vi "SCMP - Main Program v2.vi"() -> ()   [LabVIEW 2014]
doc: "Goodrich Exposure Range: .05microseconds to 798.9ms\n\nLow Gain (110e-/ADU)\nHigh Gain (6.5 e-/ADU)\n\nGA1280J Trigger Modes\n0 : Internally triggered; Internally timed\n1 : Externally triggered; Internally timed\n2 : Externally triggered; Externally timed\n3 : Externally gated; Internally timed\n\nFor list of camera commands\nsee Appendix A in the manual\n\n\nUse this template to build a standard state machine design pattern. Each state executes code and determines which state to transition to. Contrast this design pattern with the User Interface Event Handler pattern, in which code executes in response to user actions. Contrast this design pattern also with the Queued Message Handler pattern, in which each message handling code can queue zero or more new messages.\nNote: This template does not contain the most recent programming guidelines recommended by National Instruments. For a complete, project-based implementation of the Standard State Machine pattern, use the Create Project dialog box instead of this template."
uses:
  Controls/Main Program States.ctl
  <vilib>/Utility/error.llb/DialogType.ctl
  Controls/SCD - Calibration Optics Filter Wheel.ctl
  Controls/SCD - EDT - Emission Line Filter Wheel.ctl
  Controls/CoMP-S Controls/Emission Line Filter Wheel.ctl
  Controls/CoMP-S Controls/Polarization Optics Filter Wheel.ctl
  Controls/Global demo.vi
  Controls/SCD - FITS Cluster.ctl
  AISAS/Controls/focus.ctl
  AISAS/Controls/Diffuser.ctl
  Controls/Globals.vi
  AISAS/Mech/AISAS Mech.lvclass
  c:/mhutar/SCMP/Ancillary/Watlow EZ-ZONE/Public/Watbus.dll
  Ancillary/Watlow EZ-ZONE/Public/Watbus.dll
  Controls/peripherals.ctl
  AISAS/Controls/motor.ctl
  Controls/Cameras select.ctl
  Controls/FITS Data type.ctl
  Controls/Cbk Data type.ctl
  Controls/Cookbook.ctl
  Controls/beaning.ctl
  Camera/Andor Neo Info.ctl
  PI/PI Control.ctl
  AISAS/Controls/Rotation.ctl
panel:
  in  "Comment":string="Test"
  in  "Observer":string="Observer"
  out "Instrument":string
  out "Main Loop":bool=TRUE
  out "Log Loop":bool=TRUE
  out "Program":bool=TRUE
  out "Version":string
  in  "AOI Width 2":i64=2560
  in  "AOI Height 2":i64=2160
  out "Latest Actions":string="\r"
  out "cbk name":string="automated_find_focus_656.cbk"
  out "Main Loop Error":errorcluster={"status"=TRUE, "code"=0, "source"=""}
  in  "Tab Control":T1(tab)
  out "Camera T Image Zoom":u16[][](graph)
  out "Histogram Graph 2":T2(graph)
  out "Timestamp 2":timestamp=timestamp(3507746192.5616717 s since 1904-01-01)
  out "Mean ADU 2":u32=7788 format="%.1f"
  out "Sharpness 2":dbl format="%.2f"
  out "Camera FITS file path 2":path
  out "Camera R Image":u16[][](graph)
  in  "PI cam3 (mm)":T3 min=0.1 max=21.0 step=0.1 format="%.1f"
  in  "PI cam2 (mm)":T3 min=0.1 max=27.0 step=0.1 format="%.1f"
  in  "Calibration Optics":T4
  in  "Size":dbl format="%.2f"
  in  "Focus":T5 min=70.0 max=152.0 format="%.2f"
  in  "Andover Filter Wheel":T6
  in  "Calibration Wheel":T7
  in  "Binning":T8
  in  "Save Data to FITS?":bool
  out "Histogram Graph":T2(graph)
  in  "Snap Images":bool
  in  "Live Preview (Andor)":bool
  in  "Exposure (s)":dbl=0.02 min=1e-05 max=10.0 step=0.001 format="%_3p"
  out "Timestamp":timestamp=timestamp(3507746192.5616717 s since 1904-01-01)
  in  "PI cam1 (mm)":T3 min=0.1 max=27.0 step=0.1 format="%.1f"
  out "Camera FITS file path":path
  in  "Emission Line Filters":T9
  in  "Set Filter Wheels":bool
  out "Mean ADU":u32=7788 format="%.1f"
  out "Sharpness":dbl format="%.2f"
  in  "Diffuser":T10=enum."In Beam"
  in  "Rotation [deg]":T11 min=0.0 max=360.0 step=1.0 format="%.1f"
  in  "Move AISAS Mechanisms":bool
  in  "Motors":bool=TRUE
  out "Camera Image":u16[][](graph)
  out "Camera T Image":u16[][](graph)
  in  "Andor Adv Settings":bool
  in  "Diffuser 2":T10=enum."In Beam"
  in  "Focus 2":T5 min=70.0 max=152.0 format="%.2f"
  in  "Rotation [deg] 2":T11 min=0.0 max=360.0 step=1.0 format="%.1f"
  in  "Size 2":dbl format="%.2f"
  in  "Save Data to FITS?":bool=TRUE
  out "Cookbook":T12=[{"Data Type"=enum."ACQUIRE DATA", "Arg 1"=0.0, "Arg 2"=0.0, "Arg 3"=path "", "Comments"=""}, {"Data Type"=enum."ACQUIRE DATA", "Arg 1"=0.0, "Arg 2"=0.0, "Arg 3"=path "", "Comments"=""}]
  out "FITS Path from Last Recipe Acquiring Data":path
  in  "Load Cookbook":bool
  in  "Run Cookbook":bool
  out "# of Recipes":i16
  out "Selected Cookbook":path
  out "Recipe Files":string[](array[string])
  in  "limit max FPS to:":dbl=10.0 min=0.1 max=49.0 step=1.0 format="%.1g"
  out "Continually Read Log File":string="20160903-07:42:55 Live Preview Images\n20160903-07:44:38 Program Terminated\n20160903-07:45:16 Program Started\n20160903-07:45:18 Snap Single Image\n20160903-07:45:27 Live Preview Images\n20160903-07:46:17 Calibration & Filter wheel position:\t8\t5\n20160903-07:46:35 Live Preview Images\n20160903-07:50:39 Live Preview Images\n20160903-07:51:54 Camera Moved to Positon:-18.00\n20160903-07:51:55 Snap Single Image\n20160903-07:52:37 Loaded Cookbook\tfind_focus_656.cbk\n20160903-07:53:52 Run Cookbook\tfind_focus_656.cbk\n20160903-07:53:52 Recipe#0-exposure-20ms.rcp\n20160903-07:53:52 Recipe#1-fw-656.rcp\n20160903-07:53:54 Recipe#2-cal-open.rcp\n20160903-07:53:56 Recipe#3-move-absolute-neg19.rcp\n20160903-07:53:56 Recipe#4-take_656_focus_image.rcp\n20160903-07:54:02 Recipe#5-move-relative-neg0pt25.rcp\n20160903-07:55:56 Program Started\n20160903-07:56:02 Camera Moved to Positon:-18.00\n20160903-07:56:03 Snap Single Image\n20160903-07:56:35 Camera Moved to Positon:-19.00\n20160903-07:56:37 Snap Single Image\n20160903-07:56:58 Camera Moved to Positon:-20.00\n20160903-07:57:02 Snap Single Image\n20160903-07:57:20 Camera Moved to Positon:-21.00\n20160903-07:57:23 Snap Single Image\n20160903-07:57:36 Camera Moved to Positon:-22.00\n20160903-07:57:37 Snap Single Image\n20160903-07:57:53 Camera Moved to Positon:-25.00\n20160903-07:57:57 Snap Single Image\n20160903-07:58:13 Camera Moved to Positon:-30.00\n20160903-07:58:17 Snap Single Image\n20160903-07:58:43 Camera Moved to Positon:-18.00\n20160903-07:58:44 Snap Single Image\n20160903-07:58:58 Camera Moved to Positon:-17.00\n20160903-07:59:00 Snap Single Image\n20160903-08:00:39 Calibration & Filter wheel position:\t7\t6\n20160903-08:00:48 Snap Single Image\n20160903-08:01:42 Camera Moved to Positon:-65.00\n20160903-08:01:47 Snap Single Image\n20160903-08:02:07 Camera Moved to Positon:-70.00\n20160903-08:02:10 Snap Single Image\n20160903-08:02:51 Camera Moved to Positon:-75.00\n20160903-08:02:53 Snap Single Image\n20160903-08:03:25 Calibration & Filter wheel position:\t7\t7\n20160903-08:03:37 Snap Single Image\n20160903-08:03:55 Camera Moved to Positon:-76.00\n20160903-08:04:01 Snap Single Image\n20160903-08:04:13 Camera Moved to Positon:-77.00\n20160903-08:04:14 Snap Single Image\n20160903-08:04:24 Camera Moved to Positon:-78.00\n20160903-08:04:26 Snap Single Image\n20160903-08:04:38 Camera Moved to Positon:-79.00\n20160903-08:04:39 Snap Single Image\n20160903-08:04:50 Camera Moved to Positon:-83.00\n20160903-08:04:52 Snap Single Image\n20160903-08:05:10 Camera Moved to Positon:-73.00\n20160903-08:05:11 Snap Single Image\n20160903-08:05:22 Camera Moved to Positon:-71.00\n20160903-08:05:24 Snap Single Image\n20160903-08:05:34 Camera Moved to Positon:-69.00\n20160903-08:05:35 Snap Single Image\n20160903-08:05:47 Camera Moved to Positon:-67.00\n20160903-08:05:48 Snap Single Image\n20160903-08:06:13 Calibration & Filter wheel position:\t7\t8\n20160903-08:07:06 Snap Single Image\n20160903-08:07:17 Camera Moved to Positon:-69.00\n20160903-08:07:18 Snap Single Image\n20160903-08:07:28 Camera Moved to Positon:-71.00\n20160903-08:07:30 Snap Single Image\n20160903-08:07:40 Camera Moved to Positon:-73.00\n20160903-08:07:43 Snap Single Image\n20160903-08:07:53 Camera Moved to Positon:-75.00\n20160903-08:07:55 Snap Single Image\n20160903-08:08:04 Camera Moved to Positon:-77.00\n20160903-08:08:06 Snap Single Image\n20160903-08:08:17 Camera Moved to Positon:-79.00\n20160903-08:08:28 Snap Single Image\n20160903-08:08:43 Camera Moved to Positon:-81.00\n20160903-08:08:46 Snap Single Image\n20160903-08:09:05 Calibration & Filter wheel position:\t7\t9\n20160903-08:09:48 Camera Moved to Positon:-100.00\n20160903-08:09:50 Snap Single Image\n20160903-08:10:09 Snap Single Image\n20160903-08:10:26 Camera Moved to Positon:-100.00\n20160903-08:10:35 Camera Moved to Positon:-100.00\n20160903-08:10:37 Snap Single Image\n20160903-08:10:54 Camera Moved to Positon:-100.00\n20160903-08:10:59 Program Terminated\n20160903-08:12:25 Program Started\n20160903-08:12:33 Camera Moved to Positon:-100.00\n20160903-08:12:38 Program Terminated\n20160903-08:13:25 Program Started\n20160903-08:13:30 Camera Moved to Positon:-100.00\n20160903-08:13:37 Program Terminated\n20160903-08:14:12 Program Started\n20160903-08:14:19 Camera Moved to Positon:-100.00\n20160903-08:14:22 Snap Single Image\n20160903-08:14:37 Calibration & Filter wheel position:\t7\t9\n20160903-08:14:45 Snap Single Image\n20160903-08:14:56 Camera Moved to Positon:-105.00\n20160903-08:14:57 Snap Single Image\n20160903-08:15:10 Camera Moved to Positon:-110.00\n20160903-08:15:11 Snap Single Image\n20160903-08:15:23 Camera Moved to Positon:-115.00\n20160903-08:15:27 Snap Single Image\n20160903-08:15:39 Camera Moved to Positon:-120.00\n20160903-08:15:40 Snap Single Image\n20160903-08:15:59 Snap Single Image\n20160903-08:16:10 Camera Moved to Positon:-115.00\n20160903-08:16:11 Snap Single Image\n20160903-08:16:21 Camera Moved to Positon:-110.00\n20160903-08:16:22 Snap Single Image\n20160903-08:16:33 Camera Moved to Positon:-105.00\n20160903-08:16:36 Snap Single Image\n20160903-08:16:49 Camera Moved to Positon:-100.00\n20160903-08:16:51 Snap Single Image\n20160903-08:17:03 Camera Moved to Positon:-95.00\n20160903-08:17:05 Snap Single Image\n20160903-08:17:16 Camera Moved to Positon:-90.00\n20160903-08:17:18 Snap Single Image\n20160903-08:17:46 Camera Moved to Positon:-85.00\n20160903-08:17:49 Snap Single Image\n20160903-08:18:00 Camera Moved to Positon:-80.00\n20160903-08:18:02 Snap Single Image\n20160903-08:18:40 Calibration & Filter wheel position:\t7\t4\n20160903-08:18:59 Camera Moved to Positon:-20.00\n20160903-08:19:11 Snap Single Image\n20160903-08:19:23 Camera Moved to Positon:-18.00\n20160903-08:19:25 Snap Single Image\n20160903-08:19:38 Camera Moved to Positon:-22.00\n20160903-08:19:39 Snap Single Image\n20160903-08:19:51 Camera Moved to Positon:-24.00\n20160903-08:19:52 Snap Single Image\n20160903-08:20:04 Calibration & Filter wheel position:\t7\t3\n20160903-08:20:11 Snap Single Image\n20160903-08:20:22 Camera Moved to Positon:-18.00\n20160903-08:20:24 Snap Single Image\n20160903-08:20:39 Camera Moved to Positon:-16.00\n20160903-08:20:40 Snap Single Image\n20160903-08:20:53 Camera Moved to Positon:-14.00\n20160903-08:20:56 Snap Single Image\n20160903-08:21:06 Camera Moved to Positon:-12.00\n20160903-08:21:07 Snap Single Image\n20160903-08:21:16 Camera Moved to Positon:-10.00\n20160903-08:21:24 Snap Single Image\n20160903-08:21:34 Camera Moved to Positon: -8.00\n20160903-08:21:36 Snap Single Image\n20160903-08:22:12 Camera Moved to Positon: -6.00\n20160903-08:22:21 Snap Single Image\n20160903-08:23:09 Calibration & Filter wheel position:\t7\t1\n20160903-08:23:17 Snap Single Image\n20160903-08:23:27 Camera Moved to Positon: -4.00\n20160903-08:23:29 Snap Single Image\n20160903-08:23:37 Camera Moved to Positon: -2.00\n20160903-08:23:38 Snap Single Image\n20160903-08:23:47 Camera Moved to Positon:  0.00\n20160903-08:23:50 Snap Single Image\n20160903-08:26:00 Camera Moved to Positon:-18.00\n20160903-08:26:44 Program Started\n20160903-08:26:59 Camera Moved to Positon:-18.00\n20160903-08:27:05 Loaded Cookbook\tfind_focus_656.cbk\n20160903-08:27:12 Run Cookbook\tfind_focus_656.cbk\n20160903-08:27:12 Recipe#0-exposure-20ms.rcp\n20160903-08:27:12 Recipe#1-fw-656.rcp\n20160903-08:27:14 Recipe#2-cal-open.rcp\n20160903-08:27:16 Recipe#3-take_656_focus_image.rcp\n20160903-08:29:11 Camera Moved to Positon:-19.00\n20160903-08:29:17 Run Cookbook\tfind_focus_656.cbk\n20160903-08:29:17 Recipe#0-exposure-20ms.rcp\n20160903-08:29:17 Recipe#1-fw-656.rcp\n20160903-08:29:19 Recipe#2-cal-open.rcp\n20160903-08:29:21 Recipe#3-take_656_focus_image.rcp\n20160903-08:29:59 Camera Moved to Positon:-20.00\n20160903-08:30:03 Run Cookbook\tfind_focus_656.cbk\n20160903-08:30:03 Recipe#0-exposure-20ms.rcp\n20160903-08:30:03 Recipe#1-fw-656.rcp\n20160903-08:30:05 Recipe#2-cal-open.rcp\n20160903-08:30:07 Recipe#3-take_656_focus_image.rcp\n20160903-08:30:28 Camera Moved to Positon:-21.00\n20160903-08:30:32 Run Cookbook\tfind_focus_656.cbk\n20160903-08:30:32 Recipe#0-exposure-20ms.rcp\n20160903-08:30:32 Recipe#1-fw-656.rcp\n20160903-08:30:34 Recipe#2-cal-open.rcp\n20160903-08:30:36 Recipe#3-take_656_focus_image.rcp\n20160903-08:31:03 Camera Moved to Positon:-22.00\n20160903-08:31:06 Run Cookbook\tfind_focus_656.cbk\n20160903-08:31:06 Recipe#0-exposure-20ms.rcp\n20160903-08:31:06 Recipe#1-fw-656.rcp\n20160903-08:31:08 Recipe#2-cal-open.rcp\n20160903-08:31:10 Recipe#3-take_656_focus_image.rcp\n20160903-08:31:33 Camera Moved to Positon:-23.00\n20160903-08:31:38 Run Cookbook\tfind_focus_656.cbk\n20160903-08:31:38 Recipe#0-exposure-20ms.rcp\n20160903-08:31:38 Recipe#1-fw-656.rcp\n20160903-08:31:40 Recipe#2-cal-open.rcp\n20160903-08:31:42 Recipe#3-take_656_focus_image.rcp\n20160903-08:32:05 Camera Moved to Positon:-24.00\n20160903-08:32:08 Run Cookbook\tfind_focus_656.cbk\n20160903-08:32:08 Recipe#0-exposure-20ms.rcp\n20160903-08:32:08 Recipe#1-fw-656.rcp\n20160903-08:32:10 Recipe#2-cal-open.rcp\n20160903-08:32:12 Recipe#3-take_656_focus_image.rcp\n20160903-08:32:35 Camera Moved to Positon:-25.00\n20160903-08:32:40 Run Cookbook\tfind_focus_656.cbk\n20160903-08:32:40 Recipe#0-exposure-20ms.rcp\n20160903-08:32:40 Recipe#1-fw-656.rcp\n20160903-08:32:42 Recipe#2-cal-open.rcp\n20160903-08:32:44 Recipe#3-take_656_focus_image.rcp\n20160903-08:33:03 Camera Moved to Positon:-26.00\n20160903-08:33:07 Run Cookbook\tfind_focus_656.cbk\n20160903-08:33:07 Recipe#0-exposure-20ms.rcp\n20160903-08:33:07 Recipe#1-fw-656.rcp\n20160903-08:33:09 Recipe#2-cal-open.rcp\n20160903-08:33:11 Recipe#3-take_656_focus_image.rcp\n20160903-08:33:32 Camera Moved to Positon:-27.00\n20160903-08:33:34 Run Cookbook\tfind_focus_656.cbk\n20160903-08:33:34 Recipe#0-exposure-20ms.rcp\n20160903-08:33:34 Recipe#1-fw-656.rcp\n20160903-08:33:36 Recipe#2-cal-open.rcp\n20160903-08:33:38 Recipe#3-take_656_focus_image.rcp\n20160903-08:34:01 Camera Moved to Positon:-28.00\n20160903-08:34:05 Run Cookbook\tfind_focus_656.cbk\n20160903-08:34:05 Recipe#0-exposure-20ms.rcp\n20160903-08:34:05 Recipe#1-fw-656.rcp\n20160903-08:34:07 Recipe#2-cal-open.rcp\n20160903-08:34:09 Recipe#3-take_656_focus_image.rcp\n20160903-08:36:44 Camera Moved to Positon:-85.00\n20160903-08:36:51 Loaded Cookbook\tfind_focus_1083.cbk\n20160903-08:37:11 Loaded Cookbook\tfind_focus_1083.cbk\n20160903-08:37:20 Run Cookbook\tfind_focus_1083.cbk\n20160903-08:37:20 Recipe#0-exposure-120ms.rcp\n20160903-08:37:20 Recipe#1-fw-1083.rcp\n20160903-08:37:22 Recipe#2-cal-open.rcp\n20160903-08:37:23 Recipe#3-take_1083_focus_image.rcp\n20160903-08:38:05 Camera Moved to Positon:-86.00\n20160903-08:38:11 Run Cookbook\tfind_focus_1083.cbk\n20160903-08:38:11 Recipe#0-exposure-120ms.rcp\n20160903-08:38:11 Recipe#1-fw-1083.rcp\n20160903-08:38:13 Recipe#2-cal-open.rcp\n20160903-08:38:15 Recipe#3-take_1083_focus_image.rcp\n20160903-08:38:39 Camera Moved to Positon:-87.00\n20160903-08:38:43 Run Cookbook\tfind_focus_1083.cbk\n20160903-08:38:43 Recipe#0-exposure-120ms.rcp\n20160903-08:38:43 Recipe#1-fw-1083.rcp\n20160903-08:38:45 Recipe#2-cal-open.rcp\n20160903-08:38:47 Recipe#3-take_1083_focus_image.rcp\n20160903-08:39:05 Camera Moved to Positon:-88.00\n20160903-08:39:09 Run Cookbook\tfind_focus_1083.cbk\n20160903-08:39:10 Recipe#0-exposure-120ms.rcp\n20160903-08:39:10 Recipe#1-fw-1083.rcp\n20160903-08:39:12 Recipe#2-cal-open.rcp\n20160903-08:39:13 Recipe#3-take_1083_focus_image.rcp\n20160903-08:43:45 Snap Single Image\n20160903-08:43:56 Run Cookbook\tfind_focus_1083.cbk\n20160903-08:43:56 Recipe#0-exposure-120ms.rcp\n20160903-08:43:56 Recipe#1-fw-1083.rcp\n20160903-08:43:58 Recipe#2-cal-open.rcp\n20160903-08:44:00 Recipe#3-take_1083_focus_image.rcp\n20160903-08:44:24 Camera Moved to Positon:-90.00\n20160903-08:44:32 Camera Moved to Positon:-89.00\n20160903-08:44:36 Run Cookbook\tfind_focus_1083.cbk\n20160903-08:44:36 Recipe#0-exposure-120ms.rcp\n20160903-08:44:36 Recipe#1-fw-1083.rcp\n20160903-08:44:38 Recipe#2-cal-open.rcp\n20160903-08:44:40 Recipe#3-take_1083_focus_image.rcp\n20160903-08:45:03 Camera Moved to Positon:-90.00\n20160903-08:45:11 Run Cookbook\tfind_focus_1083.cbk\n20160903-08:45:12 Recipe#0-exposure-120ms.rcp\n20160903-08:45:12 Recipe#1-fw-1083.rcp\n20160903-08:45:14 Recipe#2-cal-open.rcp\n20160903-08:45:15 Recipe#3-take_1083_focus_image.rcp\n20160903-08:45:38 Camera Moved to Positon:-91.00\n20160903-08:45:41 Run Cookbook\tfind_focus_1083.cbk\n20160903-08:45:41 Recipe#0-exposure-120ms.rcp\n20160903-08:45:42 Recipe#1-fw-1083.rcp\n20160903-08:45:43 Recipe#2-cal-open.rcp\n20160903-08:45:45 Recipe#3-take_1083_focus_image.rcp\n20160903-08:46:07 Camera Moved to Positon:-92.00\n20160903-08:46:12 Run Cookbook\tfind_focus_1083.cbk\n20160903-08:46:12 Recipe#0-exposure-120ms.rcp\n20160903-08:46:12 Recipe#1-fw-1083.rcp\n20160903-08:46:14 Recipe#2-cal-open.rcp\n20160903-08:46:16 Recipe#3-take_1083_focus_image.rcp\n20160903-08:46:53 Camera Moved to Positon:-93.00\n20160903-08:46:56 Run Cookbook\tfind_focus_1083.cbk\n20160903-08:46:56 Recipe#0-exposure-120ms.rcp\n20160903-08:46:56 Recipe#1-fw-1083.rcp\n20160903-08:46:58 Recipe#2-cal-open.rcp\n20160903-08:47:00 Recipe#3-take_1083_focus_image.rcp\n20160903-08:48:13 Calibration & Filter wheel position:\t7\t3\n20160903-08:51:11 Camera Moved to Positon:-10.00\n20160903-08:51:19 Camera Moved to Positon: -5.00\n20160903-08:51:20 Live Preview Images\n20160903-08:51:43 Loaded Cookbook\tfind_focus_589.cbk\n20160903-08:52:08 Loaded Cookbook\tfocus-656.cbk\n20160903-08:52:09 Run Cookbook\tfocus-656.cbk\n20160903-08:52:09 Recipe#0-fw-656.rcp\n20160903-08:52:11 Recipe#1-cal-clear.rcp\n20160903-08:52:13 Recipe#2-exposure-200ms.rcp\n20160903-08:52:13 Recipe#3-focus-656.rcp\n20160903-08:52:24 Program Started\n20160903-08:52:33 Loaded Cookbook\tfocus-656.cbk\n20160903-08:52:40 Camera Moved to Positon: -5.00\n20160903-08:52:46 Loaded Cookbook\tfind_focus_589.cbk\n20160903-08:52:48 Run Cookbook\tfind_focus_589.cbk\n20160903-08:52:48 Recipe#0-exposure-20ms.rcp\n20160903-08:52:48 Recipe#1-fw-589.rcp\n20160903-08:52:50 Recipe#2-cal-open.rcp\n20160903-08:52:52 Recipe#3-take_589_focus_image.rcp\n20160903-08:54:55 Run Cookbook\tfind_focus_589.cbk\n20160903-08:54:55 Recipe#0-exposure-20ms.rcp\n20160903-08:54:56 Recipe#1-fw-589.rcp\n20160903-08:54:57 Recipe#2-cal-open.rcp\n20160903-08:54:59 Recipe#3-take_589_focus_image.rcp\n20160903-08:55:19 Live Preview Images\n20160903-08:56:01 Camera Moved to Positon: -6.00\n20160903-08:56:04 Run Cookbook\tfind_focus_589.cbk\n20160903-08:56:04 Recipe#0-exposure-20ms.rcp\n20160903-08:56:04 Recipe#1-fw-589.rcp\n20160903-08:56:06 Recipe#2-cal-open.rcp\n20160903-08:56:08 Recipe#3-take_589_focus_image.rcp\n20160903-08:56:40 Camera Moved to Positon: -7.00\n20160903-08:58:30 Run Cookbook\tfind_focus_589.cbk\n20160903-08:58:30 Recipe#0-exposure-20ms.rcp\n20160903-08:58:30 Recipe#1-fw-589.rcp\n20160903-08:58:32 Recipe#2-cal-open.rcp\n20160903-08:58:34 Recipe#3-take_589_focus_image.rcp\n20160903-08:59:22 Camera Moved to Positon: -8.00\n20160903-09:14:18 Program Terminated\n20160903-09:40:55 Program Started\n20160903-09:44:03 Loaded Cookbook\tautomated_find_focus_656.cbk\n20160903-09:44:43 Loaded Cookbook\tautomated_find_focus_656.cbk\n20160903-09:44:57 Run Cookbook\tautomated_find_focus_656.cbk\n20160903-09:44:57 Recipe#0-exposure-20ms.rcp\n20160903-09:44:57 Recipe#1-fw-656.rcp\n20160903-09:44:59 Recipe#2-cal-open.rcp\n20160903-09:45:01 Recipe#3-move-absolute-neg15.rcp\n20160903-09:45:02 Recipe#4-take_656_focus_image.rcp\n20160903-09:45:16 Recipe#5-move-relative-neg0pt25.rcp\n20160903-09:45:17 Recipe#6-take_656_focus_image.rcp\n20160903-09:45:31 Recipe#7-move-relative-neg0pt25.rcp\n20160903-09:45:32 Recipe#8-take_656_focus_image.rcp\n20160903-09:45:46 Recipe#9-move-relative-neg0pt25.rcp\n20160903-09:45:47 Recipe#10-take_656_focus_image.rcp\n20160903-09:46:01 Recipe#11-move-relative-neg0pt25.rcp\n20160903-09:46:02 Recipe#12-take_656_focus_image.rcp\n20160903-09:46:17 Recipe#13-move-relative-neg0pt25.rcp\n20160903-09:46:18 Recipe#14-take_656_focus_image.rcp\n20160903-09:46:32 Recipe#15-move-relative-neg0pt25.rcp\n20160903-09:46:33 Recipe#16-take_656_focus_image.rcp\n20160903-09:46:47 Recipe#17-move-relative-neg0pt25.rcp\n20160903-09:46:48 Recipe#18-take_656_focus_image.rcp\n20160903-09:47:02 Recipe#19-move-relative-neg0pt25.rcp\n20160903-09:47:03 Recipe#20-take_656_focus_image.rcp\n20160903-09:47:17 Recipe#21-move-relative-neg0pt25.rcp\n20160903-09:47:17 Recipe#22-take_656_focus_image.rcp\n20160903-09:47:32 Recipe#23-move-relative-neg0pt25.rcp\n20160903-09:47:32 Recipe#24-take_656_focus_image.rcp\n20160903-09:47:46 Recipe#25-move-relative-neg0pt25.rcp\n20160903-09:47:47 Recipe#26-take_656_focus_image.rcp\n20160903-09:48:02 Recipe#27-move-relative-neg0pt25.rcp\n20160903-09:48:03 Recipe#28-take_656_focus_image.rcp\n20160903-09:48:17 Recipe#29-move-relative-neg0pt25.rcp\n20160903-09:48:17 Recipe#30-take_656_focus_image.rcp\n20160903-09:48:32 Recipe#31-move-relative-neg0pt25.rcp\n20160903-09:48:33 Recipe#32-take_656_focus_image.rcp\n20160903-09:48:49 Recipe#33-move-relative-neg0pt25.rcp\n20160903-09:48:49 Recipe#34-take_656_focus_image.rcp\n20160903-09:49:05 Recipe#35-move-relative-neg0pt25.rcp\n20160903-09:49:06 Recipe#36-take_656_focus_image.rcp\n20160903-09:49:23 Recipe#37-move-relative-neg0pt25.rcp\n20160903-09:49:24 Recipe#38-take_656_focus_image.rcp\n20160903-09:49:41 Recipe#39-move-relative-neg0pt25.rcp\n20160903-09:49:42 Recipe#40-take_656_focus_image.rcp\n20160903-09:50:01 Recipe#41-move-relative-neg0pt25.rcp\n20160903-09:50:01 Recipe#42-take_656_focus_image.rcp\n20160903-09:50:20 Recipe#43-move-relative-neg0pt25.rcp\n20160903-09:50:21 Recipe#44-take_656_focus_image.rcp\n20160903-09:54:36 Loaded Cookbook\tautomated_find_focus_656.cbk\n20160903-09:54:47 Loaded Cookbook\tautomated_find_focus_656.cbk\n20160903-09:55:40 Loaded Cookbook\tautomated_find_focus_656.cbk\n20160903-09:55:54 Run Cookbook\tautomated_find_focus_656.cbk\n20160903-09:55:54 Recipe#0-exposure-40ms.rcp\n20160903-09:55:54 Recipe#1-fw-656.rcp\n20160903-09:55:56 Recipe#2-cal-open.rcp\n20160903-09:55:58 Recipe#3-move-absolute-neg15.rcp\n20160903-09:55:59 Recipe#4-take_656_focus_image.rcp\n20160903-09:56:06 Recipe#5-move-relative-neg0pt5.rcp\n20160903-09:56:07 Recipe#6-take_656_focus_image.rcp\n20160903-09:56:14 Recipe#7-move-relative-neg0pt5.rcp\n20160903-09:56:15 Recipe#8-take_656_focus_image.rcp\n20160903-09:56:22 Recipe#9-move-relative-neg0pt5.rcp\n20160903-09:56:22 Recipe#10-take_656_focus_image.rcp\n20160903-09:56:29 Recipe#11-move-relative-neg0pt5.rcp\n20160903-09:56:30 Recipe#12-take_656_focus_image.rcp\n20160903-09:56:37 Recipe#13-move-relative-neg0pt5.rcp\n20160903-09:56:38 Recipe#14-take_656_focus_image.rcp\n20160903-09:56:45 Recipe#15-move-relative-neg0pt5.rcp\n20160903-09:56:45 Recipe#16-take_656_focus_image.rcp\n20160903-09:56:52 Recipe#17-move-relative-neg0pt5.rcp\n20160903-09:56:53 Recipe#18-take_656_focus_image.rcp\n20160903-09:57:00 Recipe#19-move-relative-neg0pt5.rcp\n20160903-09:57:01 Recipe#20-take_656_focus_image.rcp\n20160903-09:57:08 Recipe#21-move-relative-neg0pt5.rcp\n20160903-09:57:09 Recipe#22-take_656_focus_image.rcp\n20160903-09:57:16 Recipe#23-move-relative-neg0pt5.rcp\n20160903-09:57:16 Recipe#24-take_656_focus_image.rcp\n20160903-09:57:23 Recipe#25-move-relative-neg0pt5.rcp\n20160903-09:57:24 Recipe#26-take_656_focus_image.rcp\n20160903-09:57:31 Recipe#27-move-relative-neg0pt5.rcp\n20160903-09:57:32 Recipe#28-take_656_focus_image.rcp\n20160903-09:57:39 Recipe#29-move-relative-neg0pt5.rcp\n20160903-09:57:40 Recipe#30-take_656_focus_image.rcp\n20160903-09:57:47 Recipe#31-move-relative-neg0pt5.rcp\n20160903-09:57:48 Recipe#32-take_656_focus_image.rcp\n20160903-09:57:55 Recipe#33-move-relative-neg0pt5.rcp\n20160903-09:57:56 Recipe#34-take_656_focus_image.rcp\n20160903-09:58:03 Recipe#35-move-relative-neg0pt5.rcp\n20160903-09:58:03 Recipe#36-take_656_focus_image.rcp\n20160903-09:58:10 Recipe#37-move-relative-neg0pt5.rcp\n20160903-09:58:11 Recipe#38-take_656_focus_image.rcp\n20160903-09:58:18 Recipe#39-move-relative-neg0pt5.rcp\n20160903-09:58:19 Recipe#40-take_656_focus_image.rcp\n20160903-09:58:26 Recipe#41-move-relative-neg0pt5.rcp\n20160903-09:58:27 Recipe#42-take_656_focus_image.rcp\n20160903-09:58:34 Recipe#43-move-relative-neg0pt5.rcp\n20160903-09:58:35 Recipe#44-take_656_focus_image.rcp\n20160903-10:46:33 Program Terminated\n20160903-12:25:32 Program Started\n20160903-12:26:22 Program Terminated\n20160903-12:45:45 Program Started\n20160903-12:45:56 Program Terminated\n20160903-12:49:12 Program Started\n20160903-12:49:15 Loaded Cookbook\tautomated_find_focus_656.cbk\n20160903-12:49:24 Run Cookbook\tautomated_find_focus_656.cbk\n20160903-12:49:25 Recipe#0-exposure-40ms.rcp\n20160903-12:49:25 Recipe#1-fw-656.rcp\n20160903-12:49:26 Recipe#2-cal-open.rcp\n20160903-12:49:28 Recipe#3-move-absolute-neg15.rcp\n20160903-12:49:29 Recipe#4-take_656_focus_image.rcp\n20160903-12:49:32 Recipe#5-move-relative-neg0pt5.rcp\n20160903-12:49:33 Recipe#6-take_656_focus_image.rcp\n20160903-12:49:36 Recipe#7-move-relative-neg0pt5.rcp\n20160903-12:49:36 Recipe#8-take_656_focus_image.rcp\n20160903-12:49:39 Recipe#9-move-relative-neg0pt5.rcp\n20160903-12:49:40 Recipe#10-take_656_focus_image.rcp\n20160903-12:49:43 Recipe#11-move-relative-neg0pt5.rcp\n20160903-12:49:43 Recipe#12-take_656_focus_image.rcp\n20160903-12:49:46 Recipe#13-move-relative-neg0pt5.rcp\n20160903-12:49:47 Recipe#14-take_656_focus_image.rcp\n20160903-12:49:49 Recipe#15-move-relative-neg0pt5.rcp\n20160903-12:49:50 Recipe#16-take_656_focus_image.rcp\n20160903-12:49:53 Recipe#17-move-relative-neg0pt5.rcp\n20160903-12:49:53 Recipe#18-take_656_focus_image.rcp\n20160903-12:49:56 Recipe#19-move-relative-neg0pt5.rcp\n20160903-12:49:57 Recipe#20-take_656_focus_image.rcp\n20160903-12:49:59 Recipe#21-move-relative-neg0pt5.rcp\n20160903-12:50:00 Recipe#22-take_656_focus_image.rcp\n20160903-12:50:03 Recipe#23-move-relative-neg0pt5.rcp\n20160903-12:50:04 Recipe#24-take_656_focus_image.rcp\n20160903-12:50:06 Recipe#25-move-relative-neg0pt5.rcp\n20160903-12:50:07 Recipe#26-take_656_focus_image.rcp\n20160903-12:50:10 Recipe#27-move-relative-neg0pt5.rcp\n20160903-12:50:10 Recipe#28-take_656_focus_image.rcp\n20160903-12:50:13 Recipe#29-move-relative-neg0pt5.rcp\n20160903-12:50:14 Recipe#30-take_656_focus_image.rcp\n20160903-12:50:16 Recipe#31-move-relative-neg0pt5.rcp\n20160903-12:50:17 Recipe#32-take_656_focus_image.rcp\n20160903-12:50:20 Recipe#33-move-relative-neg0pt5.rcp\n20160903-12:50:20 Recipe#34-take_656_focus_image.rcp\n20160903-12:50:23 Recipe#35-move-relative-neg0pt5.rcp\n20160903-12:50:24 Recipe#36-take_656_focus_image.rcp\n20160903-12:50:26 Recipe#37-move-relative-neg0pt5.rcp\n20160903-12:50:27 Recipe#38-take_656_focus_image.rcp\n20160903-12:50:30 Recipe#39-move-relative-neg0pt5.rcp\n20160903-12:50:31 Recipe#40-take_656_focus_image.rcp\n20160903-12:50:33 Recipe#41-move-relative-neg0pt5.rcp\n20160903-12:50:34 Recipe#42-take_656_focus_image.rcp\n20160903-12:50:37 Recipe#43-move-relative-neg0pt5.rcp\n20160903-12:50:37 Recipe#44-take_656_focus_image.rcp\n20160903-13:54:17 Program Terminated\n20160903-14:07:18 Program Started\n20160903-14:08:12 Program Terminated\n20160903-14:20:46 Program Started\n20160903-14:22:56 Program Terminated\n20160903-14:23:20 Program Started\n20160903-14:25:03 Program Terminated\n20160903-14:31:16 Program Started\n20160903-14:32:59 Program Terminated\n20160903-14:33:26 Program Started\n20160903-14:35:01 Program Terminated\n20160903-14:36:43 Program Started\n20160903-14:38:01 Program Terminated\n20160903-14:39:22 Program Started\n20160903-14:39:47 Program Terminated\n20160903-14:40:22 Program Started\n20160903-14:41:59 Program Terminated\n20160903-15:07:40 Program Started\n20160903-15:10:18 Program Terminated\n20160903-15:19:59 Program Started\n20160903-15:20:17 Program Terminated\n20160903-15:20:43 Program Started\n20160903-15:20:43 Program Terminated\n20160903-15:21:33 Program Started\n20160903-15:22:45 Program Terminated\n20160903-15:24:43 Program Started\n20160903-15:26:40 Program Terminated\n20160903-15:29:07 Program Started\n20160903-15:29:52 Loaded Cookbook\tautomated_find_focus_656.cbk\n20160903-15:30:08 Loaded Cookbook\tautomated_find_focus_656.cbk\n"
  out "min Cookbook Exposure [s]":dbl=200.0 format="%#_3p"
  out "Today's SCMP Log File":path
  out "Cookbook Comments":string
  in  "Mod/Seq":bool
  in  "Enable Data Logging":bool=TRUE
  out "Today's SCMP Eng  File":path
  out "Air around \nprefilter wheel [C]":sgl(graph)
  out "Lyot Filter Temp [C]":dbl(graph)
  out "Air around Camera [C]":sgl(graph)
  out "Air around Lyot Filter [C]":dbl(graph)
  out "Eng Data Error":errorcluster={"status"=TRUE, "code"=0, "source"=""}
  out "Camera 1 Temp [C}":dbl(graph)=-21.03
  out "Camera 2 Temp [C}":dbl(graph)=-21.03
  out "FITS Header":T14={"Wavelength (nm)"=530.15, "Exposure (s)"=0.05, "Tuning Delay (ms)"=1000.0, "Beam Type (-1/1)"=1.0, "Tuning Voltages"=[1.111, 2.222, 3.333, 4.444], "Observer"="observer", "Light Shapping Diffuser"=enum."In Beam", "Comment"="", "Data Type"=9, "Mod Cycles"=0, "SCD Calibration Optics"=enum."1 - Polarizer @0, I+Q", "SCD Emission Line Filter"=enum."1-557.6nm", "Cookbook"="", "COMP-S Calibration Wheel"=enum."Dark", "COMP-S Andover Filter Wheel"=enum."530.3nm/HWB 0.34nm (Fe XIV)", "FOV Rotation (deg)"=66.0, "Objective Lens Position (mm)"=0.0, "Occulter size"=0.0, "Time End"=timestamp(3382374145.421875 s since 1904-01-01), "Acc Exposure (s)"=0.0, "Time Stamp Array"=[], "Camera Serial Number"=[], "Camera Temp"=[], "Camera PI (mm)"=[], "Time Start"=timestamp(3382374145.421875 s since 1904-01-01), "Peripherals"={"ILX controler"=FALSE, "Zone temperatures"=FALSE, "Andor"=FALSE, "Andor 2"=FALSE, "PI Stages"=FALSE, "AISAS mechanisms"=FALSE, "AISAS Mech.lvclass"=refnum, "Zone temp ref"=variant, "FWs"=FALSE}, "FITS paths"=[], "Cameras"=enum."Andor", "load preset cbk"=FALSE, "periodic check count"=0, "COMP-S Calibration Wheel 2"=enum."Dark", "Calib"=enum."Dark", "Abso Aperture"=40.0, "Nominal Aperture"=196.0} {"Nominal Aperture" format="%.1f"; "Abso Aperture" format="%.1f"; "Camera PI (mm)" format="%_3g"; "Acc Exposure (s)" format="%^.3g"; "Occulter size" format="%.2f"; "Objective Lens Position (mm)" min=70.0 max=152.0 format="%.2f"; "FOV Rotation (deg)" format="%.1f"; "Data Type" items=["LIVE", "DARK", "FLAT", "CALI", "OBSE", "ABSO", "AURE", "TARG", "OBJE", "HOLE", "OREX", "THRO", "CHIP"]; "Exposure (s)" format="%^.3g"; "Wavelength (nm)" format="%_6g"}
  out "Andor Neo":T17[](array[typedef]) {"Exposure (s)" format="%^.3g"; "Time at Synch" format="%<%H:%M:%S>T"; "Interframe Time" format="%#_3g"; "Frame Readout Time" format="%_3g"; "Row Readout Time" format="%_3g"}
  in  "Stop":bool=TRUE
  # "Filter Wheels"
  # "Camera Settings"
  # "AISAS mechanisms"
  # "Occulter"
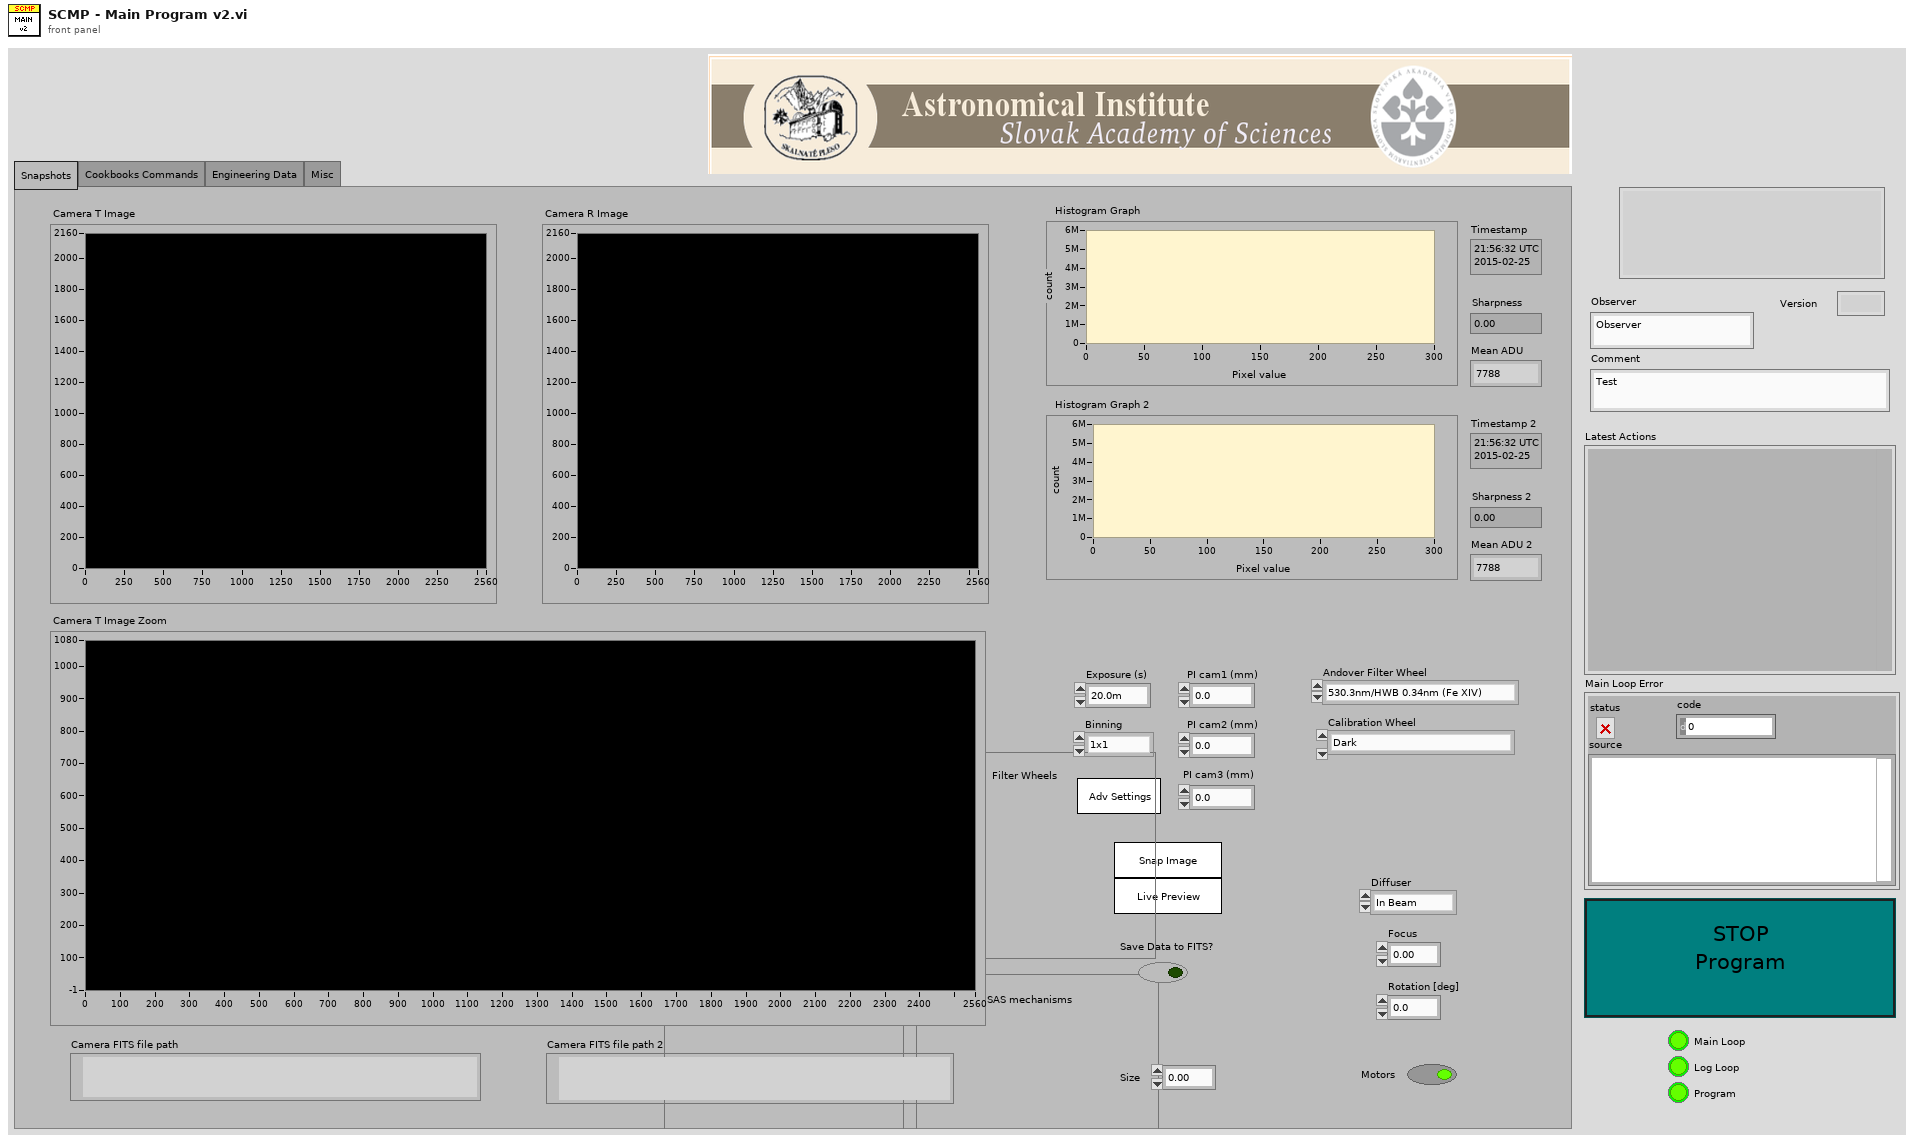
[diagram p1: front panel]
types:
  T1 = enum32{"Snapshots", "Cookbooks Commands", "Engineering Data", "Misc"}
  T2 = cluster{"X Values":dbl[], "Histogram: h(x)":i32[]}
  T3 = typedef "PI Control.ctl" = dbl
  T4 = typedef "SCD - Calibration Optics Filter Wheel.ctl" = enum16{"1 - Polarizer @0, I+Q", "2 - Polarizer @90, I-Q", "3 - Polarizer @45, I+U", "4 - Polarizer @135, I-U", "5 - Polarizer @0, Retarder @45, I+V", "6 - Polarizer @0, Retarder @135, I-V", "7 - Dark", "8 - Clear", "9 - N/A"}
  T5 = typedef "focus.ctl" = dbl
  T6 = typedef "Emission Line Filter Wheel.ctl" = enum16{"530.3nm/HWB 0.34nm (Fe XIV)", "587.6nm/HBW 0.44nm (He I D3)", "637.5nm/HBW 0.53nm (Fe X)", "656.3nm/HBW 0.57nm (H-Alpha)", "789.2nm/HBW 0.85nm (Fe XI)", "854.2nm/HBW 1.01nm (Ca I)", "1074.7nm/HBW 2.34nm (Fe XIII)", "1079.8nm/HBW 1.64nm (Fe XIII)", "1083.0nm/HBW 1.66nm (He I)"}
  T7 = typedef "Polarization Optics Filter Wheel.ctl" = enum16{"Dark", "Clear", "Exchange Lens", "Polarizer @0, I+Q", "Polarizer @90, I-Q", "Polarizer @45, I+U", "Polarizer @135, I-U", "Polarizer @0, Retarder @45, I+V", "Polarizer @0, Retarder @135, I-V"}
  T8 = typedef "beaning.ctl" = enum16{"1x1", "2x2", "3x3", "4x4", "8x8"}
  T9 = typedef "SCD - EDT - Emission Line Filter Wheel.ctl" = enum16{"1-557.6nm", "2-587.6nm", "3-589.6nm", "4-630.2nm", "5-656.4nm", "6-849.8nm", "7-854.2nm", "8-866.2nm", "9-1083.0nm"}
  T10 = typedef "Diffuser.ctl" = enum16{"Out of Beam", "In Beam"}
  T11 = typedef "Rotation.ctl" = dbl
  T12 = typedef "Cookbook.ctl" = cluster{"Data Type":T13, "Arg 1":sgl, "Arg 2":sgl, "Arg 3":path, "Comments":string}[]
  T13 = typedef "Cbk Data type.ctl" = enum32{"ACQUIRE DATA", "SET DIFFUSER", "CAL-FW", "WAVELENGTH-FW", "INSTR. ROTATION", "SET FOCUS", "DATATYPE", "SET EXPOSURE", "CBK COMMENTS", "MOVE-PI", "MOVE-PI2", "MOVE-PI3", "DWELL TIME", "BINNING"}
  T14 = typedef "SCD - FITS Cluster.ctl" = cluster{"Wavelength (nm)":dbl, "Exposure (s)":dbl, "Tuning Delay (ms)":dbl, "Beam Type (-1/1)":dbl, "Tuning Voltages":dbl[], "Observer":string, "Light Shapping Diffuser":T10, "Comment":string, "Data Type":u16, "Mod Cycles":u16, "SCD Calibration Optics":T4, "SCD Emission Line Filter":T9, "Cookbook":string, "COMP-S Calibration Wheel":T7, "COMP-S Andover Filter Wheel":T6, "FOV Rotation (deg)":dbl, "Objective Lens Position (mm)":T5, "Occulter size":dbl, "Time End":timestamp, "Acc Exposure (s)":dbl, "Time Stamp Array":timestamp[], "Camera Serial Number":string[], "Camera Temp":dbl[], "Camera PI (mm)":dbl[], "Time Start":timestamp, "Peripherals":T15, "FITS paths":path[], "Cameras":T16, "load preset cbk":bool, "periodic check count":i32, "COMP-S Calibration Wheel 2":T7, "Calib":enum16{"Dark", "Flat"}, "Abso Aperture":dbl, "Nominal Aperture":dbl}
  T15 = typedef "peripherals.ctl" = cluster{"ILX controler":bool, "Zone temperatures":bool, "Andor":bool, "Andor 2":bool, "PI Stages":bool, "AISAS mechanisms":bool, "AISAS Mech.lvclass":refnum<class "AISAS Mech.lvclass">, "Zone temp ref":variant, "FWs":bool}
  T16 = typedef "Cameras select.ctl" = enum16{"Andor", "GDR"}
  T17 = typedef "Andor Neo Info.ctl" = cluster{"Handle":i32, "Pixel Encoding":string, "AOI Width":i32, "AOI Height":i32, "AOI Stride":i32, "Row Readout Time":dbl, "Frame Readout Time":dbl, "Interframe Time":dbl, "Semaphore":T18, "SerialNumber":string, "Camera Model":string, "Controller ID":string, "Firmware Version":string, "Shutter":string, "BDiv":u8, "Time at Synch":timestamp, "Idx":i32, "PreAmp":string, "Binning":T8, "PixelReadoutRate":string, "Exposure (s)":dbl, "Image Bytes":i64, "Image Pixels":i64, "SpuriousNoiseFilter":bool, "Overlap":bool, "CycleMode":string}
  T18 = typedef "Semaphore RefNum" = refnum<k1>
  T19 = typedef "Main Program States.ctl" = enum16{"Initialize", "Wait for Event", "Periodic Check", "Update UI", "Update Camera UI", "Load Cookbook", "Run Cookbook", "Snap Images", "Live Preview", "Set Filter Wheel", "Set Calibration Wheel", "AISAS Motors on/off", "AISAS Move", "Move AISAS Mechanisms", "Stop", "Change Camera Exposure", "Change Camera Stage Position", "Set Camera AOI", "Andor Adv Settings", "Update Image", "Run Dark", "Calib acq", "Process Calib"}
  T20 = typedef "SCD - FITS Cluster.ctl" = cluster{"Wavelength (nm)":dbl, "Exposure (s)":dbl, "Tuning Delay (ms)":dbl, "Beam Type (-1/1)":dbl, "Tuning Voltages":dbl[], "Observer":string, "Light Shapping Diffuser":T10, "Comment":string, "Data Type":T21, "Mod Cycles":u16, "SCD Calibration Optics":T4, "SCD Emission Line Filter":T9, "Cookbook":string, "COMP-S Calibration Wheel":T7, "COMP-S Andover Filter Wheel":T6, "FOV Rotation (deg)":dbl, "Objective Lens Position (mm)":T5, "Occulter size":dbl, "Time End":timestamp, "Acc Exposure (s)":dbl, "Time Stamp Array":timestamp[], "Camera Serial Number":string[], "Camera Temp":dbl[], "Camera PI (mm)":dbl[], "Time Start":timestamp, "Peripherals":T15, "FITS paths":path[], "Cameras":T16, "load preset cbk":bool, "periodic check count":i32, "COMP-S Calibration Wheel 2":T7, "Calib":enum16{"Dark", "Flat"}, "Abso Aperture":dbl, "Nominal Aperture":dbl, "Pointer IP":string}
  T21 = typedef "FITS Data type.ctl" = enum16{"LIVE", "DARK", "FLAT", "CALI", "OBSE", "ABSO", "AURE", "TARG", "OBJE", "HOLE", "OREX", "THRO", "CHIP"}
  T22 = enum8{"Enabled", "Disabled", "Disabled and Grayed Out"}
  T23 = typedef "motor.ctl" = enum32{"Rotation", "Diffuser ", "Focus"}
  T24 = enum16{"Emission Line Filters", "Calibration Polarizers"}
  T25 = typedef "DialogType.ctl" = u16
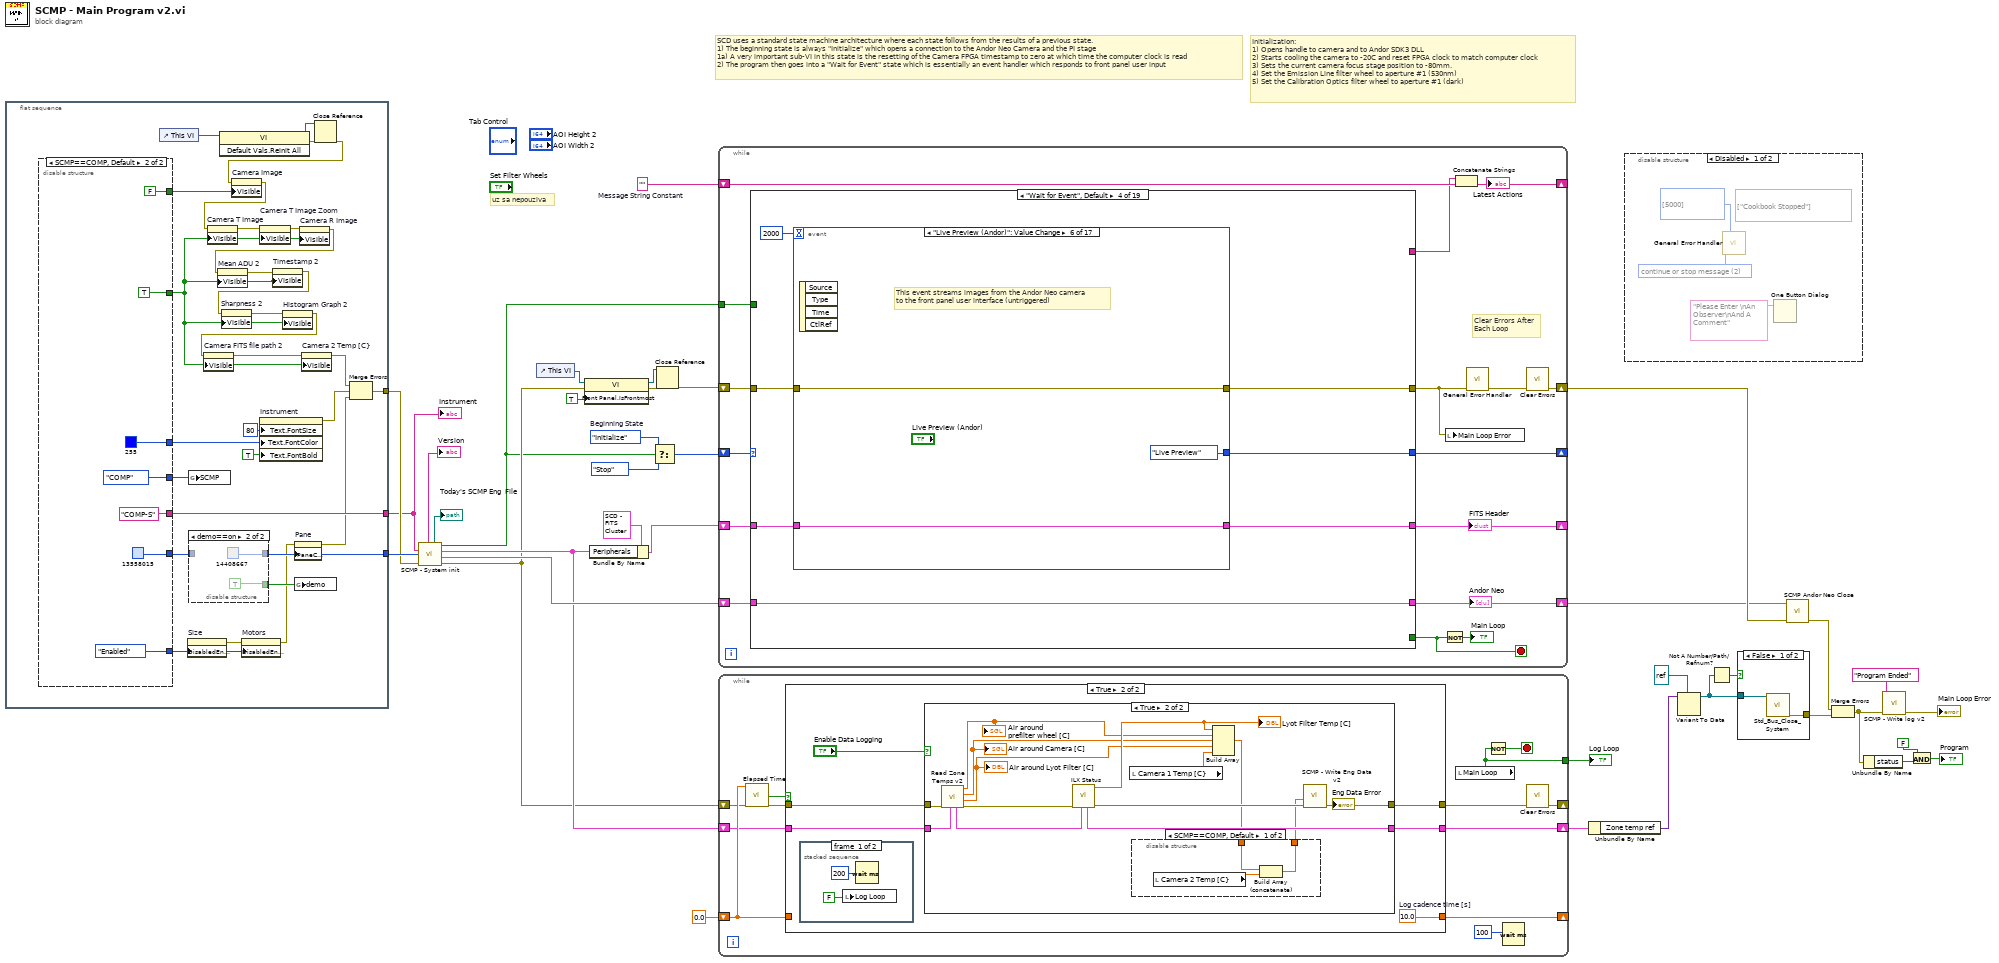
[diagram p0: block diagram]
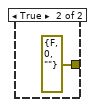
[diagram p2: hidden frame]
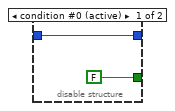
[diagram p3: hidden frame]
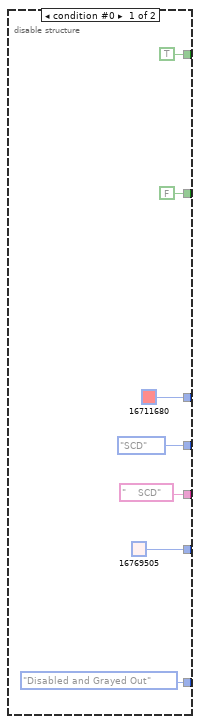
[diagram p4: hidden frame]
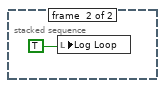
[diagram p7: hidden frame]
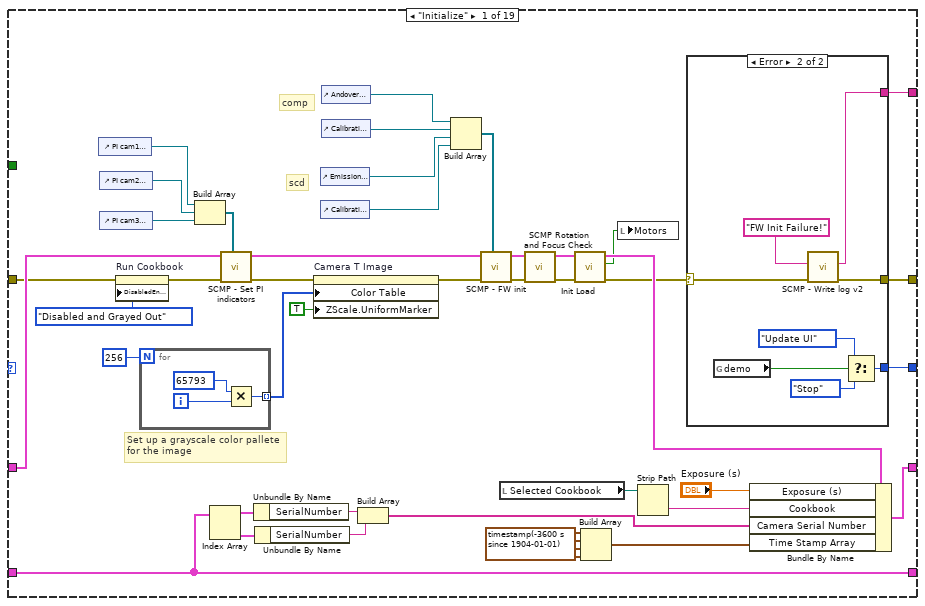
[diagram p10: hidden frame]
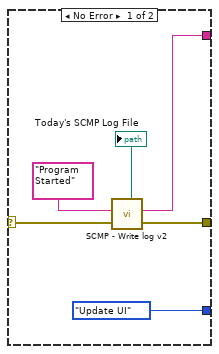
[diagram p11: hidden frame]
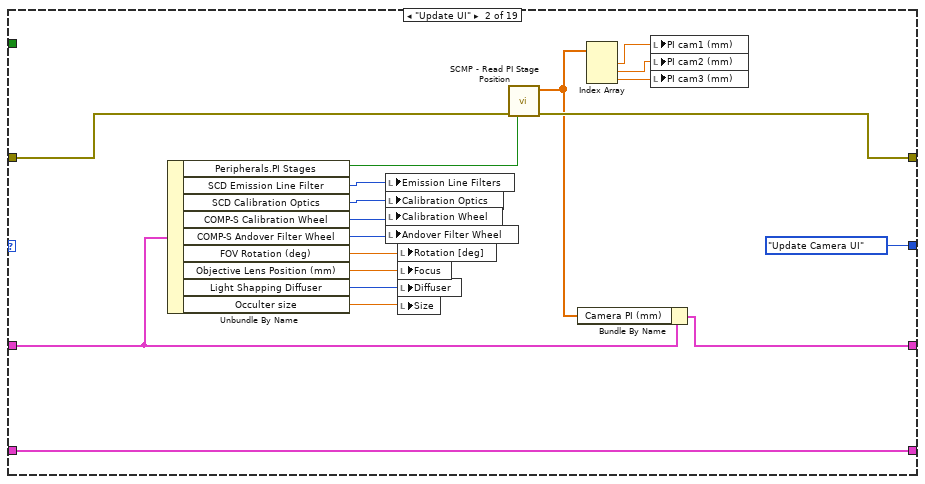
[diagram p12: hidden frame]
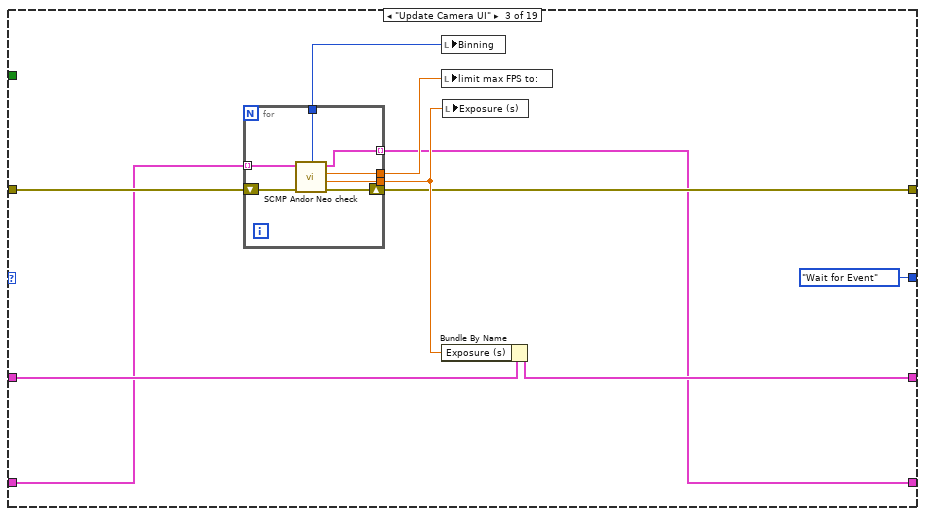
[diagram p13: hidden frame]
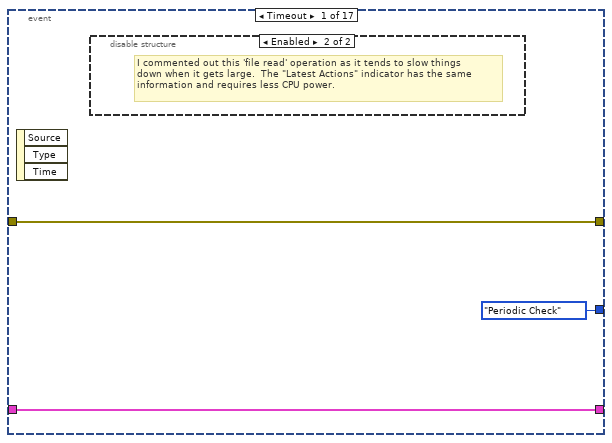
[diagram p14: hidden frame]
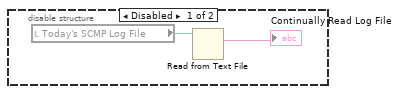
[diagram p15: hidden frame]
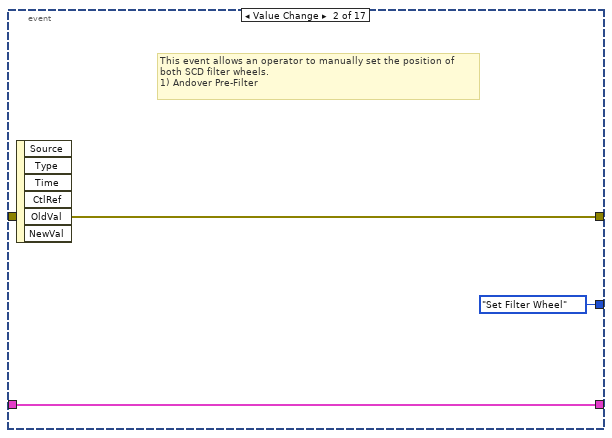
[diagram p16: hidden frame]
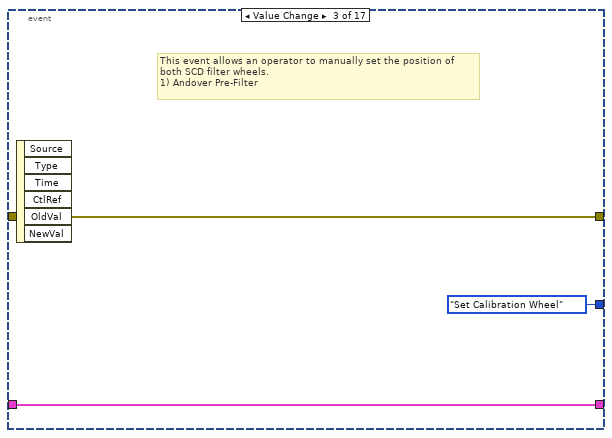
[diagram p17: hidden frame]
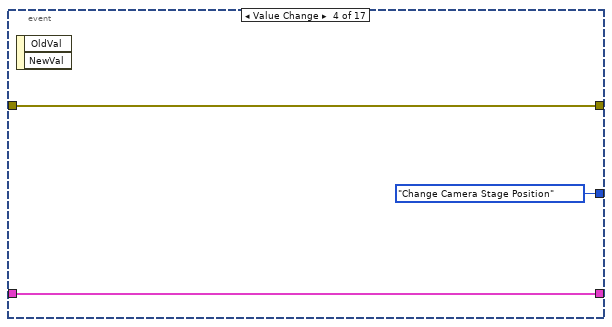
[diagram p18: hidden frame]
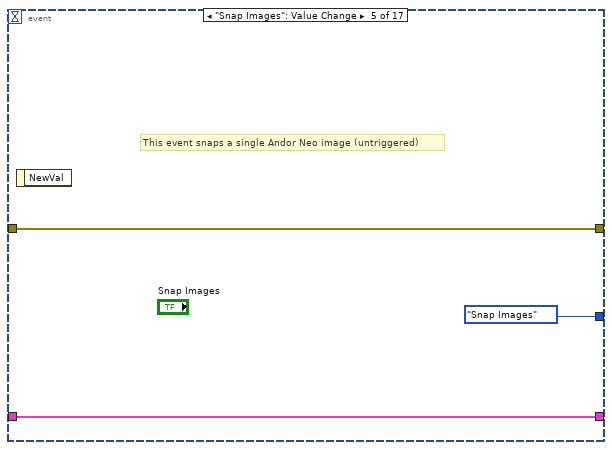
[diagram p19: hidden frame]
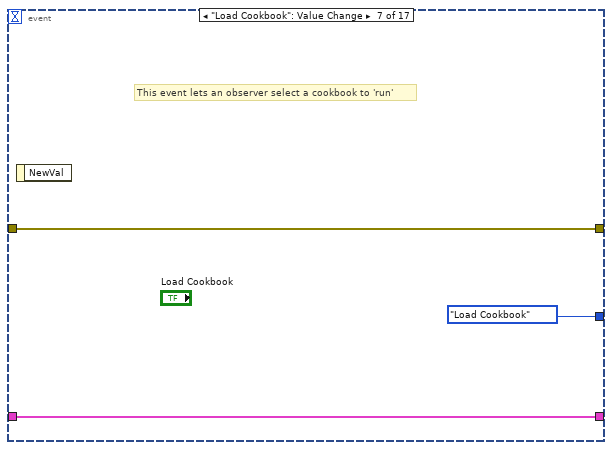
[diagram p20: hidden frame]
diagram:
  w10 = Main_Program_States."Initialize"  # Beginning State
  w37 = ""  # Message String Constant
  # "uz sa nepouziva"
  # "Initialization:\n1) Opens handle to camera and to Andor SDK3 DLL\n2) Starts cooling the camera to -20C and reset FPGA clock to match computer clock\n3) Sets the current camera focus stage position to -80mm.\n4) Set the Emission Line filter wheel to aperture #1 (530nm)\n5) Set the Calibration Optics filter wheel to aperture #1 (dark)"
  # "SCD uses a standard state machine architecture where each state follows from the results of a previous state.\n1) The beginning state is always \"Initialize\" which opens a connection to the Andor Neo Camera and the PI stage\n1a) A very important sub-VI in this state is the resetting of the Camera FPGA timestamp to zero at which time the computer clock is read\n2) The program then goes into a \"Wait for Event\" state which is essentially an event handler which responds to front panel user input"
  n1 = flat-sequence {
    tunnel: [w58] -> w17
    tunnel: [w57] -> w5
    tunnel: [w44] -> w15
    frame #0 {
      n2 = disable-structure "Conditional Disable Structure" shown="SCMP==COMP, Default" {
        disable-tunnel: [TRUE ("Visible") FALSE ("Visible")] -> w62
        disable-tunnel: ["    SCD" ("String") "COMP-S" ("String")] -> w57
        disable-tunnel: [u32 16711680 u32 255] -> w65
        disable-tunnel: [u32 16769505 u32 13558015] -> w64
        disable-tunnel: [T22."Disabled and Grayed Out" ("Disabled") T22."Enabled" ("Disabled")] -> w60
        disable-tunnel: [FALSE ("Visible") TRUE ("Visible")] -> w59
        disable-tunnel: [enum16{"COMP", "SCD"}."SCD" ("SCMP") enum16{"COMP", "SCD"}."COMP" ("SCMP")] -> w61
        frame condition #0 {
        }
        frame condition #1 (active) {
        }
      }
      n3 = control-ref of="This VI"() -> (w41:refnum<vi>)
      n4 = property on="Size" class="DigNum (strict)"("DisabledEnum"=w60) -> (error out=w56:errorcluster)  [unwired: 2 in, 1 out]
      n5 = global write "Globals.vi" "SCMP"(w61) -> ()
      n6 = disable-structure shown="demo==on" {
        disable-tunnel: [w69 u32 14408667] -> w58
        disable-tunnel: w64 -> [w69 _]
        disable-tunnel: [FALSE ("demo") TRUE ("demo")] -> w63
        frame condition #0 (active) {
        }
        frame condition #1 {
        }
      }
      n7 = invoke class="VI" method="Default Vals.Reinit All"(reference=w41) -> (reference out=w39:refnum<vi>, error out=w40:errorcluster)  [unwired: 2 in, 1 out]
      n8 = property on="Motors" class="Bool (strict)"(error in=w56, "DisabledEnum"=w60) -> (error out=w55:errorcluster)  [unwired: 1 in, 1 out]
      n9 = property on="Instrument" class="Str"("Text.FontSize"=u32 80 ("Text.Font:Color"), "Text.FontColor"=w65, "Text.FontBold"=TRUE ("Text.Font:Bold")) -> (error out=w43:errorcluster)  [unwired: 2 in, 1 out]
      n10 = property on="Pane" class="Pane"(error in=w55, "PaneColor"=w58) -> (error out=w42:errorcluster)  [unwired: 1 in, 1 out]
      n11 = global write "Global demo.vi" "demo"(w63) -> ()
      n12 = Close Reference(reference=w39, error in (no error)=w40) -> (error out=w38:errorcluster)
      n13 = property on="Camera Image" class="IntGraph (strict)"(error in=w38, "Visible"=w62) -> (error out=w46:errorcluster)  [unwired: 1 in, 1 out]
      n14 = property on="Camera T Image" class="IntGraph (strict)"(error in=w46, "Visible"=w59) -> (error out=w52:errorcluster)  [unwired: 1 in, 1 out]
      n15 = property on="Camera T Image Zoom" class="IntGraph (strict)"(error in=w52, "Visible"=w59) -> (error out=w51:errorcluster)  [unwired: 1 in, 1 out]
      n16 = property on="Camera R Image" class="IntGraph (strict)"(error in=w51, "Visible"=w59) -> (error out=w50:errorcluster)  [unwired: 1 in, 1 out]
      n17 = property on="Mean ADU 2" class="DigNum (strict)"(error in=w50, "Visible"=w59) -> (error out=w49:errorcluster)  [unwired: 1 in, 1 out]
      n18 = property on="Timestamp 2" class="AbsTime (strict)"(error in=w49, "Visible"=w59) -> (error out=w48:errorcluster)  [unwired: 1 in, 1 out]
      n19 = property on="Sharpness 2" class="DigNum (strict)"(error in=w48, "Visible"=w59) -> (error out=w47:errorcluster)  [unwired: 1 in, 1 out]
      n20 = property on="Histogram Graph 2" class="XYGraph (strict)"(error in=w47, "Visible"=w59) -> (error out=w53:errorcluster)  [unwired: 1 in, 1 out]
      n21 = property on="Camera FITS file path 2" class="Path"(error in=w53, "Visible"=w59) -> (error out=w54:errorcluster)  [unwired: 1 in, 1 out]
      n22 = property on="Camera 2 Temp [C}" class="WFChart (strict)"(error in=w54, "Visible"=w59) -> (error out=w45:errorcluster)  [unwired: 1 in, 1 out]
      n23 = Merge Errors(w45, w43, w42) -> (w44:errorcluster)
    }
  }
  n24 = call "SCMP - System init.vi"("error in (no error)"=w15, "Pane Color"=w17, "instrument"=w5) -> ("error main"=w11:errorcluster, "Andor array"=w20:T17[], "Peripherals"=w19:T15, "cont?"=w7:bool, "Today's SCMP Engineering File"=→"Today's SCMP Eng  File":path, "version"=→"Version":string)  [unwired: 3 in]
  n25 = control-ref of="This VI"() -> (w16:refnum<vi>)
  n26 = property class="VI"(reference=w16, error in=w11, "Front Panel.IsFrontmost"=TRUE ("Front Panel Window:Is Frontmost")) -> (reference out=w13:refnum<vi>, error out=w14:errorcluster)
  n27 = Bundle By Name(cluster=T20 {"Wavelength (nm)"=530.15, "Exposure (s)"=0.05, "Tuning Delay (ms)"=200.0, "Beam Type (-1/1)"=1.0, "Tuning Voltages"=[1.111, 2.222, 3.333, 4.444], "Observer"="observer", "Light Shapping Diffuser"=enum."In Beam", "Comment"="", "Data Type"=enum."LIVE", "Mod Cycles"=1, "SCD Calibration Optics"=enum."1 - Polarizer @0, I+Q", "SCD Emission Line Filter"=enum."1-557.6nm", "Cookbook"="", "COMP-S Calibration Wheel"=enum."Dark", "COMP-S Andover Filter Wheel"=enum."530.3nm/HWB 0.34nm (Fe XIV)", "FOV Rotation (deg)"=66.0, "Objective Lens Position (mm)"=0.0, "Occulter size"=0.0, "Time End"=timestamp(3382374145.421875 s since 1904-01-01), "Acc Exposure (s)"=0.0, "Time Stamp Array"=[], "Camera Serial Number"=[], "Camera Temp"=[], "Camera PI (mm)"=[0.0, 0.0, 0.0], "Time Start"=timestamp(3382374145.421875 s since 1904-01-01), "Peripherals"={"ILX controler"=FALSE, "Zone temperatures"=FALSE, "Andor"=FALSE, "Andor 2"=FALSE, "PI Stages"=FALSE, "AISAS mechanisms"=FALSE, "AISAS Mech.lvclass"=refnum, "Zone temp ref"=variant, "FWs"=FALSE}, "FITS paths"=[], "Cameras"=enum."Andor", "load preset cbk"=FALSE, "periodic check count"=0, "COMP-S Calibration Wheel 2"=enum."Dark", "Calib"=enum."Dark", "Abso Aperture"=40.0, "Nominal Aperture"=196.0, "Pointer IP"="127.0.0.1"} ("FITS"), "Peripherals"=w19) -> (w23:T20)
  n28 = Select(t=w10, s=w7, f=Main_Program_States."Stop" ("Beginning State")) -> (s? t:f=w8:T19)
  n29 = Close Reference(reference=w13, error in (no error)=w14) -> (error out=w12:errorcluster)
  n30 = while {
    shift-right: [w95] -> w33
    shift-left: w12 -> [w101]
    shift-right: [w96] -> _
    shift-left: w37 -> [w98]
    shift-right: [w90] -> _
    shift-left: w23 -> [w100]
    shift-right: [w91] -> w25
    shift-left: w20 -> [w99]
    shift-right: [w88] -> _
    shift-left: w8 -> [w89]
    tunnel: w7 -> [w86]
    stop <- w87 stop-if-true
    # "Clear Errors After\nEach Loop"
    n31 = case shown="\"Wait for Event\", Default" w89 {
      tunnel: [w128 Main_Program_States."Update Camera UI" ("Next State") Main_Program_States."Wait for Event" ("Next State") w196 Main_Program_States."Wait for Event" ("Next State") Main_Program_States."Wait for Event" ("Next State") Main_Program_States."Update UI" ("Beginning State") Main_Program_States."Wait for Event" ("Next State") Main_Program_States."Update UI" ("Beginning State") Main_Program_States."Wait for Event" ("Next State") Main_Program_States."Wait for Event" ("Next State") Main_Program_States."Wait for Event" ("Next State") Main_Program_States."Update UI" ("Next State") w538 Main_Program_States."Update UI" ("Next State") Main_Program_States."Update Camera UI" ("Beginning State") Main_Program_States."Update Camera UI" ("Beginning State") Main_Program_States."Update Camera UI" ("Beginning State") Main_Program_States."Stop" ("Next State")] -> w88
      tunnel: w101 -> [w103 w165 w186 w200 w285 w333 w349 w362 w400 w436 w463 w492 w517 w533 w600 w623 w646 w669 w682]
      tunnel: [w142 w163 w182 w199 w291 w332 w352 w360 w422 w434 w462 w491 w502 w535 w596 w622 w641 w668 w683] -> w92
      tunnel: [w132 _ _ _ w288 w334 w351 w371 w395 w438 w465 w490 w519 w537 w601 w624 w643 _ w685] -> w97
      tunnel: w100 -> [w111 w162 w188 w198 w287 w311 w347 w370 w416 w430 w458 w487 w518 w532 w590 w629 w647 w665 w675]
      tunnel: [w130 w160 w187 w197 w281 w311 w346 w369 w403 w429 w457 w486 w501 w534 w597 w629 w647 w665 w675] -> w90
      tunnel: w99 -> [w131 w177 w181 w201 w290 w328 w345 w358 w417 w437 w464 w500 w522 w536 w598 w618 w638 w664 w684]
      tunnel: [w131 w177 w180 w201 w290 w328 w345 w358 w417 w437 w464 w500 w522 w536 w598 w618 w637 w664 w684] -> w91
      tunnel: [_ _ _ _ _ _ _ _ _ _ _ _ _ _ _ _ _ _ TRUE ("x = y?")] -> w87
      tunnel: w86 -> [_ _ _ _ _ _ _ _ _ _ _ _ _ _ _ _ _ _ w672]
      frame "Initialize" {
        w137 = timestamp(-3600 s since 1904-01-01) ("element")
        # "Set up a grayscale color pallete for the image"
        # "scd"
        # "comp"
        n32 = control-ref of="PI cam1 (mm)"() -> (w113:refnum<vi>)
        n33 = control-ref of="PI cam2 (mm)"() -> (w114:refnum<vi>)
        n34 = control-ref of="PI cam3 (mm)"() -> (w115:refnum<vi>)
        n35 = property on="Run Cookbook" class="Bool"(error in=w103, "DisabledEnum"=T22."Disabled and Grayed Out" ("Disabled")) -> (error out=w102:errorcluster)  [unwired: 1 in, 1 out]
        n36 = for {
          N: 256 -> [_]
          tunnel: [w144] -> w108 mode=indexing
          i -> [w145]
          n37 = Multiply(x=65793, y=w145) -> (x*y=w144:i32)
        }
        n38 = Build Array(w113, w114, w115) -> (w112:refnum<vi>[])
        n39 = Index Array(array=w131) -> (element #1=w136:T17, element #2=w134:T17)  [unwired: 2 in]
        n40 = call "SCMP - Set PI indicators.vi"("PI refs"=w112, "error in (no error)"=w102, "FITS Header in"=w111) -> ("error out"=w107:errorcluster, "FITS Header out"=w110:T20)  [unwired: 7 in]
        n41 = Unbundle By Name(w136) -> ("SerialNumber"=w135:string)
        n42 = Unbundle By Name(w134) -> ("SerialNumber"=w133:string)
        n43 = property on="Camera T Image" class="IntGraph (strict)"(error in=w107, "Color Table"=w108, "ZScale.UniformMarker"=TRUE ("Z Scale.Uniform Marker Spacing?")) -> (error out=w106:errorcluster)  [unwired: 1 in, 1 out]
        n44 = control-ref of="Emission Line Filters"() -> (w119:refnum<vi>)
        n45 = control-ref of="Calibration Optics"() -> (w118:refnum<vi>)
        n46 = control-ref of="Andover Filter Wheel"() -> (w121:refnum<vi>)
        n47 = control-ref of="Calibration Wheel"() -> (w120:refnum<vi>)
        n48 = Build Array(w135, w133) -> (w123:string[])
        n49 = Build Array(w121, w120, w119, w118) -> (w117:refnum<vi>[])
        n50 = call "SCMP - FW init.vi"("FW refs"=w117, "error in (no error)"=w106, "FITS Header in"=w110) -> ("error out"=w139:errorcluster, "FITS Header out"=w127:T20)  [unwired: 7 in]
        n51 = local read "Selected Cookbook"() -> (w141:path)
        n52 = call "SCMP Rotation and Focus Check.vi"("error in"=w139, "FITS Header In"=w127) -> ("error out"=w129:errorcluster, "FITS Header Out"=w126:T20)  [unwired: 5 in, 3 out]
        n53 = call "Init Load.vi"("error in (no error)"=w129, "FITS Header in"=w126) -> ("error out"=w116:errorcluster, "Motors (off/on)"=w124:bool, "FITS Header out"=w125:T20)  [unwired: 7 in]
        n54 = Build Array(w137, w137, w137, w137) -> (w122:timestamp[])
        n55 = local write "Motors"(w124) -> ()
        n56 = Strip Path(path=w141) -> (name=w140:string)  [unwired: 1 out]
        n57 = case shown="Error" w116 {
          selector: w116 -> [w149 w159]
          tunnel: [w147 w156] -> w132
          tunnel: [w148 w158] -> w142
          tunnel: [Main_Program_States."Update UI" ("Beginning State") w152] -> w128
          frame No Error {
            n58 = call "SCMP - Write log v2.vi"("Error to log"=w149, "data"="Program Started") -> ("error out"=w148:errorcluster, "Last Log Entry"=w147:string, "Today's SCMP Log File"=→"Today's SCMP Log File":path)  [unwired: 7 in]
          }
          frame Error {
            n59 = global read "Global demo.vi" "demo"() -> (w153:bool)
            n60 = call "SCMP - Write log v2.vi"("Error to log"=w159, "data"="FW Init Failure!") -> ("error out"=w158:errorcluster, "Last Log Entry"=w156:string)  [unwired: 7 in, 1 out]
            n61 = Select(t=Main_Program_States."Update UI" ("Beginning State"), s=w153, f=Main_Program_States."Stop" ("Beginning State")) -> (s? t:f=w152:T19)
          }
        }
        n62 = Bundle By Name(cluster=w125, "Exposure (s)"="Exposure (s)", "Cookbook"=w140, "Camera Serial Number"=w123, "Time Stamp Array"=w122) -> (w130:T20)
      }
      frame "Update UI" {
        n63 = Unbundle By Name(w162) -> ("Peripherals.PI Stages"=w164:bool, "SCD Emission Line Filter"=w166:T9, "SCD Calibration Optics"=w167:T4, "COMP-S Calibration Wheel"=w168:T7, "COMP-S Andover Filter Wheel"=w169:T6, "FOV Rotation (deg)"=w170:dbl, "Objective Lens Position (mm)"=w171:T5, "Light Shapping Diffuser"=w172:T10, "Occulter size"=w173:dbl)
        n64 = local write "Emission Line Filters"(w166) -> ()
        n65 = local write "Calibration Optics"(w167) -> ()
        n66 = local write "Calibration Wheel"(w168) -> ()
        n67 = local write "Andover Filter Wheel"(w169) -> ()
        n68 = local write "Rotation [deg]"(w170) -> ()
        n69 = local write "Focus"(w171) -> ()
        n70 = local write "Diffuser"(w172) -> ()
        n71 = local write "Size"(w173) -> ()
        n72 = call "SCMP - Read PI Stage Position.vi"("Enable"=w164, "error in (no error)"=w165) -> ("error out"=w163:errorcluster, "Output Array"=w161:dbl[])  [unwired: 8 in]
        n73 = Bundle By Name(cluster=w162, "Camera PI (mm)"=w161) -> (w160:T20)
        n74 = Index Array(array=w161) -> (element #1=w174:dbl, element #2=w175:dbl, element #3=w176:dbl)  [unwired: 3 in]
        n75 = local write "PI cam1 (mm)"(w174) -> ()
        n76 = local write "PI cam2 (mm)"(w175) -> ()
        n77 = local write "PI cam3 (mm)"(w176) -> ()
      }
      frame "Update Camera UI" {
        n78 = for {
          tunnel: [w194] -> w185
          tunnel: [w193] -> w184
          tunnel: [w192] -> w183
          shift-right: [w191] -> w182
          shift-left: w186 -> [w195]
          tunnel: w181 -> [w190] mode=indexing
          tunnel: [w189] -> w180 mode=indexing
          n79 = call "SCMP Andor Neo check.vi"("error in"=w195, "Andor"=w190) -> ("error out"=w191:errorcluster, "Exp"=w192:dbl, "FPS"=w193:dbl, "Andor out"=w189:T17, "binning"=w194:u8)  [unwired: 5 in]
        }
        n80 = local write "Binning"(w185) -> ()
        n81 = local write "limit max FPS to:"(w184) -> ()
        n82 = Bundle By Name(cluster=w188, "Exposure (s)"=w183) -> (w187:T20)
        n83 = local write "Exposure (s)"(w183) -> ()
      }
      frame "Wait for Event", Default {
        n84 = event shown="[5] \"Live Preview (Andor)\": Value Change" {
          selector: _ -> [_ _ _ _ _ _ _ _ _ _ _ _ _ _ _ _ _]
          dyn-events: _ -> [_ _ _ _ _ _ _ _ _ _ _ _ _ _ _ _ _]
          timeout: 2000 -> [_ _ _ _ _ _ _ _ _ _ _ _ _ _ _ _ _]
          tunnel: [Main_Program_States."Periodic Check" ("Next State") Main_Program_States."Set Filter Wheel" ("Next State") Main_Program_States."Set Calibration Wheel" ("Next State") Main_Program_States."Change Camera Stage Position" ("Next State") Main_Program_States."Snap Images" ("Next State") Main_Program_States."Live Preview" ("Next State") Main_Program_States."Load Cookbook" ("Next State") Main_Program_States."Run Cookbook" ("Next State") Main_Program_States."Move AISAS Mechanisms" ("Next State") Main_Program_States."AISAS Motors on/off" ("Next State") Main_Program_States."AISAS Move" ("Next State") Main_Program_States."AISAS Move" ("Next State") Main_Program_States."AISAS Move" ("Next State") Main_Program_States."Change Camera Exposure" ("Next State") Main_Program_States."Set Camera AOI" ("Next State") Main_Program_States."Andor Adv Settings" ("Next State") Main_Program_States."Stop" ("Next State")] -> w196
          tunnel: w200 -> [w205 w210 w213 w215 w218 w222 w224 w227 w230 w233 w244 w254 w264 w266 w269 w272 w275]
          tunnel: [w205 w210 w213 w215 w218 w222 w224 w227 w230 w233 w242 w252 w262 w266 w269 w272 w275] -> w199
          tunnel: w198 -> [w204 w209 w212 w214 w217 w221 w223 w226 w229 w232 w241 w251 w261 w265 w268 w271 w274]
          tunnel: [w204 w209 w212 w214 w217 w221 w223 w226 w229 w232 w239 w249 w259 w265 w268 w271 w274] -> w197
          event Timeout {
            n85 = event-data() -> ()  [unwired: 1 in, 3 out]
            n86 = disable-structure shown="Enabled" {
              frame Disabled {
                n87 = local read "Today's SCMP Log File"() -> (w207:path)
                n88 = Read from Text File(file (use dialog)=w207) -> (text=→"Continually Read Log File":string)  [unwired: 3 in, 3 out]
              }
              frame Enabled {
                # "I commented out this 'file read' operation as it tends to slow things\ndown when it gets large.  The \"Latest Actions\" indicator has the same\ninformation and requires less CPU power."
              }
            }
          }
          event Value Change {
            # "This event allows an operator to manually set the position of\nboth SCD filter wheels.  \n1) Andover Pre-Filter"
            n89 = event-data() -> ()  [unwired: 1 in, 6 out]
          }
          event Value Change {
            # "This event allows an operator to manually set the position of\nboth SCD filter wheels.  \n1) Andover Pre-Filter"
            n90 = event-data() -> ()  [unwired: 1 in, 6 out]
          }
          event Value Change {
            n91 = event-data() -> ()  [unwired: 1 in, 2 out]
          }
          event "Snap Images": Value Change {
            # "This event snaps a single Andor Neo image (untriggered)"
            n92 = event-data() -> ()  [unwired: 1 in, 1 out]
          }
          event "Live Preview (Andor)": Value Change {
            # "This event streams images from the Andor Neo camera\nto the front panel user interface (untriggered)"
            n93 = event-data() -> ()  [unwired: 1 in, 4 out]
          }
          event "Load Cookbook": Value Change {
            # "This event lets an observer select a cookbook to 'run'"
            n94 = event-data() -> ()  [unwired: 1 in, 1 out]
          }
          event "Run Cookbook": Value Change {
            # "This event runs a previously loaded cookbook sequence\nCookbooks can take many minutes to run..."
            n95 = event-data() -> ()  [unwired: 1 in, 1 out]
          }
          event "Move AISAS Mechanisms": Value Change {
            n96 = event-data() -> ()  [unwired: 1 in, 2 out]
          }
          event "Motors": Value Change {
            n97 = event-data() -> ()  [unwired: 1 in, 2 out]
          }
          event Value Change {
            n98 = event-data() -> ()  [unwired: 1 in, 6 out]
            n99 = Unbundle By Name(w241) -> ("Peripherals.AISAS Mech.lvclass"=w243:refnum<class "AISAS Mech.lvclass">)
            n100 = To Variant(anything="Diffuser") -> (Variant=w238:variant)
            n101 = call "Write Move Motor.vi"("error in (no error)"=w244, "Desired Value"=w238, "Motor"=motor."Diffuser ", "AISAS Mech in"=w243) -> ("error out"=w242:errorcluster, "AISAS Mech out"=w240:refnum<class "AISAS Mech.lvclass">)  [unwired: 6 in]
            n102 = Bundle By Name(cluster=w241, "Peripherals.AISAS Mech.lvclass"=w240) -> (w239:T20)
          }
          event Value Change {
            n103 = event-data() -> ()  [unwired: 1 in, 6 out]
            n104 = Unbundle By Name(w251) -> ("Peripherals.AISAS Mech.lvclass"=w253:refnum<class "AISAS Mech.lvclass">)
            n105 = To Variant(anything="Rotation [deg]") -> (Variant=w248:variant)
            n106 = call "Write Move Motor.vi"("error in (no error)"=w254, "Desired Value"=w248, "Motor"=motor."Rotation", "AISAS Mech in"=w253) -> ("error out"=w252:errorcluster, "AISAS Mech out"=w250:refnum<class "AISAS Mech.lvclass">)  [unwired: 6 in]
            n107 = Bundle By Name(cluster=w251, "Peripherals.AISAS Mech.lvclass"=w250) -> (w249:T20)
          }
          event Value Change {
            n108 = event-data() -> ()  [unwired: 1 in, 6 out]
            n109 = Unbundle By Name(w261) -> ("Peripherals.AISAS Mech.lvclass"=w263:refnum<class "AISAS Mech.lvclass">)
            n110 = To Variant(anything="Focus") -> (Variant=w258:variant)
            n111 = call "Write Move Motor.vi"("error in (no error)"=w264, "Desired Value"=w258, "Motor"=motor."Focus", "AISAS Mech in"=w263) -> ("error out"=w262:errorcluster, "AISAS Mech out"=w260:refnum<class "AISAS Mech.lvclass">)  [unwired: 6 in]
            n112 = Bundle By Name(cluster=w261, "Peripherals.AISAS Mech.lvclass"=w260) -> (w259:T20)
          }
          event "Exposure (s)": Value Change {
            n113 = event-data() -> ()  [unwired: 1 in, 2 out]
          }
          event Value Change {
            n114 = event-data() -> ()  [unwired: 1 in, 3 out]
          }
          event "Andor Adv Settings": Value Change {
            n115 = event-data() -> ()  [unwired: 1 in, 2 out]
          }
          event "Stop": Value Change {
            # "This event causes the SCD program to terminate"
            n116 = event-data() -> ()  [unwired: 1 in, 1 out]
          }
        }
      }
      frame "Periodic Check" {
        # "funkcia AISAS auto off:\nvypnutie tlac. Motors v pripade chyby"
        # "2sec interval (po event timeout case)"
        n117 = call "Camera temp.vi"("error in (no error)"=w285, "Andor Neo"=w290) -> ("error out"=w293:errorcluster, "Camera 2 Temp [C}"=w294:dbl, "Camera 1 Temp [C}"=w295:dbl)  [unwired: 7 in]
        "Camera 1 Temp [C}" <- w295
        "Camera 2 Temp [C}" <- w294
        n118 = Build Array(w295, w294) -> (w286:dbl[])
        n119 = Bundle By Name(cluster=w287, "Observer"="Observer", "Comment"="Comment", "Camera Temp"=w286, "Occulter size"="Size") -> (w283:T20)
        n120 = Unbundle By Name(w283) -> ("Peripherals"=w284:T15)
        n121 = call "Check.vi"("Peripherals in"=w284, "error in (no error)"=w293) -> ("error out"=w279:errorcluster, "auto off?"=w277:bool, "Peripherals out"=w282:T15, "auto off resp"=w292:string)  [unwired: 5 in, 1 out]
        n122 = Bundle By Name(cluster=w283, "Peripherals"=w282) -> (w281:T20)
        n123 = case shown="True" w277 {
          tunnel: w279 -> [w298 w299]
          tunnel: [w298 w301] -> w278
          frame False {
          }
          frame True {
            n124 = property on="Motors" class="Bool (strict)"("Val(Sgnl)"=FALSE ("Value (Signaling)")) -> (error out=w300:errorcluster)  [unwired: 2 in, 1 out]
            n125 = Merge Errors(w299, w300) -> (w301:errorcluster)
          }
        }
        n126 = case shown="Error" w278 {
          selector: w278 -> [w304 w305]
          tunnel: [w304 w309] -> w291
          tunnel: w292 -> [_ w306]
          tunnel: ["" ("Last Log Entry") w308] -> w288
          frame No Error {
          }
          frame Error {
            n127 = call "SCMP - Write log v2.vi"("Error to log"=w305, "data to end"=w306, "data"="AISAS Check ") -> ("error out"=w309:errorcluster, "Last Log Entry"=w308:string)  [unwired: 6 in, 1 out]
          }
        }
      }
      frame "Snap Images" {
        n128 = local read "Save Data to FITS?"() -> (w329:bool)
        n129 = Bundle By Name(cluster=w311, "Wavelength (nm)"=0.0) -> (w310:T20)
        n130 = call "SCMP - Snap Single Image.vi"("FITS Header"=w310, "error in"=w333, "Andor Neo"=w328, "Save Data to FITS? (F)"=w329) -> ("error out"=w331:errorcluster, "Image Graph 2"=w325:u16[][], "Image Graph"=w314:u16[][], "Snapshot FITS arr"=w326:path[], "FPGA Timestamp arr"=w327:timestamp[])  [unwired: 3 in]
        n131 = call "SCD - Determine Image Sharpness from 2D Derivative.vi"("Image In"=w314) -> ("Sharpness"=→"Sharpness":dbl)  [unwired: 9 in, 1 out]
        n132 = Index Array(array=w327) -> (element #1=→"Timestamp":timestamp, element #2=→"Timestamp 2":timestamp)  [unwired: 2 in]
        n133 = call "Neo - Calculate Image Statistics and Histogram2.vi"("Image In"=w314) -> ("Histogram Graph"=→"Histogram Graph":T2, "Mean ADU"=→"Mean ADU":dbl)  [unwired: 8 in, 1 out]
        n134 = call "Neo - Calculate Image Statistics and Histogram2.vi"("Image In"=w325) -> ("Histogram Graph"=→"Histogram Graph 2":T2, "Mean ADU"=→"Mean ADU 2":dbl)  [unwired: 8 in, 1 out]
        n135 = call "SCD - Determine Image Sharpness from 2D Derivative.vi"("Image In"=w325) -> ("Sharpness"=→"Sharpness 2":dbl)  [unwired: 9 in, 1 out]
        n136 = Index Array(array=w326) -> (element #1=→"Camera FITS file path":path, element #2=→"Camera FITS file path 2":path)  [unwired: 2 in]
        n137 = Array Size(array=w314) -> (size(s)=w313:i32[])
        n138 = Index Array(array=w313) -> (element=w312:i32)  [unwired: 1 in]
        n139 = disable-structure shown="SCMP==COMP, Default" {
          disable-tunnel: w314 -> [w342 w343]
          disable-tunnel: w325 -> [w341 _]
          disable-tunnel: w312 -> [w337 _]
          frame condition #0 (active) {
            n140 = property on="Camera R Image" class="IntGraph (strict)"("YScale.Maximum"=w337) -> (error out=w338:errorcluster)  [unwired: 2 in, 1 out]
            n141 = Divide(x=w337, y=2) -> (x/y=w339:dbl)
            n142 = property on="Camera T Image Zoom" class="IntGraph (strict)"("YScale.Maximum"=w339) -> ()  [unwired: 2 in, 2 out]
            n143 = property on="Camera T Image" class="IntGraph (strict)"(error in=w338, "YScale.Maximum"=w337) -> ()  [unwired: 1 in, 2 out]
            "Camera T Image Zoom" <- w342
            "Camera R Image" <- w341
            "Camera T Image" <- w342
          }
          frame condition #1 {
            "Camera Image" <- w343
          }
        }
        n144 = call "SCMP - Write log v2.vi"("Error to log"=w331, "data"="Snap Single Image") -> ("error out"=w332:errorcluster, "Last Log Entry"=w334:string)  [unwired: 7 in, 1 out]
      }
      frame "Live Preview" {
        n145 = call "SCMP - Live preview (ext trigger).vi"("FITS Header in"=w347, "error in"=w349, "Andor Neo"=w345, "Save Data? (F)"="Save Data to FITS?") -> ("error out"=w350:errorcluster, "FITS Header out"=w346:T14)  [unwired: 6 in]
        n146 = call "SCMP - Write log v2.vi"("Error to log"=w350, "data"="Live Preview Images") -> ("error out"=w352:errorcluster, "Last Log Entry"=w351:string)  [unwired: 7 in, 1 out]
      }
      frame "Load Cookbook" {
        n147 = call "SCMP - Read Cookbook.vi"("error in"=w362) -> ("error out"=w356:errorcluster, "Recipe Files"=→"Recipe Files":string[], "# of Recipes"=w364:i16, "Cookbook"=→"Cookbook":T12, "min Cookbook Exposure [s]"=w355:dbl, "Selected Cookbook"=w359:path, "Cookbook Comments"=→"Cookbook Comments":string)  [unwired: 4 in]
        "Selected Cookbook" <- w359
        "min Cookbook Exposure [s]" <- w355
        n148 = Greater Than 0?(x=w355) -> (x > 0?=w354:bool)
        n149 = Index Array(array=w358) -> (element=w357:T17)  [unwired: 1 in]
        n150 = case shown="True" w354 {
          tunnel: w357 -> [_ w376]
          tunnel: w355 -> [_ w374]
          frame False {
          }
          frame True {
            n151 = call "SCMP - Set Exp and Check FPS.vi"("Andor"=w376, "Set Exp or Check Fps (Set Exp)"=enum16{"Set Exp", "Check FPS"}."Check FPS", "Exposure [s]"=w374) -> ("FPS"=w377:dbl)  [unwired: 7 in, 1 out]
            n152 = local write "limit max FPS to:"(w377) -> ()
          }
        }
        n153 = case shown="No Error" w356 {
          selector: w356 -> [w382 w388]
          tunnel: w364 -> [w385 _]
          tunnel: w359 -> [w383 w391]
          tunnel: [w384 w389] -> w372
          tunnel: [w382 w388] -> w367
          frame No Error {
            n154 = Strip Path(path=w383) -> (name=w380:string)  [unwired: 1 out]
            "cbk name" <- w380
            n155 = property on="Run Cookbook" class="Bool"("DisabledEnum"=T22."Enabled" ("Disabled")) -> ()  [unwired: 2 in, 2 out]
            n156 = Concatenate Strings("Loaded Cookbook" ("data"), "\t", w380) -> (w384:string)
            "# of Recipes" <- w385
          }
          frame Error {
            n157 = Strip Path(path=w391) -> (name=w390:string)  [unwired: 1 out]
            n158 = Concatenate Strings("Error Loading Cookbook" ("data"), "\t", w390) -> (w389:string)
            n159 = property on="Run Cookbook" class="Bool"("DisabledEnum"=T22."Disabled and Grayed Out" ("Disabled")) -> ()  [unwired: 2 in, 2 out]
          }
        }
        n160 = Strip Path(path=w359) -> (name=w368:string)  [unwired: 1 out]
        n161 = Bundle By Name(cluster=w370, "Cookbook"=w368) -> (w369:T20)
        n162 = call "SCMP - Write log v2.vi"("Error to log"=w367, "data"=w372) -> ("error out"=w361:errorcluster, "Last Log Entry"=w371:string)  [unwired: 7 in, 1 out]
        n163 = call <vilib>:"Clear Errors.vi"("error in (no error)"=w361) -> ("error out"=w360:errorcluster)  [unwired: 5 in, 1 out]
      }
      frame "Run Cookbook" {
        n164 = local read "cbk name"() -> (w396:string)
        n165 = Concatenate Strings("Run Cookbook" ("data"), "\t", w396) -> (w401:string)
        n166 = call "SCMP - Write log v2.vi"("Error to log"=w400, "data"=w401) -> ("error out"=w399:errorcluster, "Last Log Entry"=w393:string)  [unwired: 7 in, 1 out]
        n167 = flat-sequence {
          tunnel: [w427] -> w413
          tunnel: w399 -> [w427]
          tunnel: [w426] -> w409
          frame #0 {
            n168 = Get Date/Time In Seconds() -> (seconds since 1Jan1904=w426:timestamp)
          }
        }
        n169 = local read "Cookbook"() -> (w419:T12)
        n170 = local read "Motors"() -> (w415:bool)
        n171 = call "SCMP - Run Cookbook.vi"("Cookbook"=w419, "Mod/Seq"="Mod/Seq", "Save to FITS?"="Save Data to FITS?", "limit max FPS to:"="limit max FPS to:", "Motors"=w415, "Error in"=w413, "Andor Neo"=w417, "FITS Header In"=w416) -> ("Result"=w407:string, "FITS Path Out"=→"FITS Path from Last Recipe Acquiring Data":path, "Updated Header"=w403:T14, "Error out"=w412:errorcluster)  [unwired: 4 in]
        n172 = flat-sequence {
          tunnel: [w425] -> w411
          tunnel: w412 -> [w425]
          tunnel: [w424] -> w410
          frame #0 {
            n173 = Get Date/Time In Seconds() -> (seconds since 1Jan1904=w424:timestamp)
          }
        }
        n174 = Subtract(x=w410, y=w409) -> (x-y=w408:dbl)
        n175 = Format Date/Time String(time format string (%c)="%M:%S] ", seconds (now)=w408) -> (date/time string=w405:string)  [unwired: 1 in]
        n176 = Concatenate Strings(w407, " [" ("string"), w405) -> (w423:string)
        n177 = call "SCMP - Write log v2.vi"("Error to log"=w411, "data"=w423) -> ("error out"=w422:errorcluster, "Last Log Entry"=w394:string)  [unwired: 7 in, 1 out]
        n178 = Concatenate Strings(w394, w393) -> (w395:string)
      }
      frame "Set Filter Wheel" {
        n179 = disable-structure shown="SCMP==COMP, Default" {
          disable-tunnel: w436 -> [w448 w455]
          disable-tunnel: [w447 w454] -> w435
          disable-tunnel: [w441 w449] -> w433
          disable-tunnel: [w445 w453] -> w429
          disable-tunnel: w430 -> [w446 w452]
          frame condition #0 {
            n180 = disable-structure shown="Disabled" {
              frame Disabled {
                # "old filter wheel vi"
                n181 = call "Optec IFW3 - Standalone.vi"() -> ()  [unwired: 11 in, 1 out]
              }
              frame Enabled {
              }
            }
            n182 = call "SCD - wavelenght.vi"("SCD Emission Line Filter"="Emission Line Filters") -> ("Numeric"=w442:dbl)  [unwired: 10 in]
            n183 = call "Optec IFW3 - Set Position with Error Handling.vi"("error in"=w448, "Emission Line Filter"="Emission Line Filters", "Filter Wheel Selector"=T24."Emission Line Filters") -> ("error out"=w441:errorcluster, "Actual Position (1-9)"=w447:i32)  [unwired: 6 in, 1 out]
            n184 = Bundle By Name(cluster=w446, "SCD Emission Line Filter"="Emission Line Filters", "Wavelength (nm)"=w442) -> (w445:T20)
          }
          frame condition #1 (active) {
            n185 = call "COMP - wavelenght.vi"("COMP-S Andover Filter Wheel"="Andover Filter Wheel") -> ("Wavelength (nm)"=w450:dbl)  [unwired: 10 in]
            n186 = call "CoMP-S Mechanism - FW.vi"("error in (no error)"=w455, "Emission Line Filters [530.3 nm]"="Andover Filter Wheel", "Filter Wheel Selector"=T24."Emission Line Filters") -> ("error out"=w449:errorcluster, "Position"=w454:i32)  [unwired: 5 in, 2 out]
            n187 = Bundle By Name(cluster=w452, "COMP-S Andover Filter Wheel"="Andover Filter Wheel", "Wavelength (nm)"=w450) -> (w453:T20)
          }
        }
        n188 = Number To Decimal String(number=w435) -> (decimal integer string=w431:string)  [unwired: 1 in]
        n189 = Concatenate Strings("Updated Filter Wheel to position:" ("data"), "\t", w431) -> (w432:string)
        n190 = call "SCMP - Write log v2.vi"("Error to log"=w433, "data"=w432) -> ("error out"=w434:errorcluster, "Last Log Entry"=w438:string)  [unwired: 7 in, 1 out]
      }
      frame "Set Calibration Wheel" {
        n191 = disable-structure shown="SCMP==COMP, Default" {
          disable-tunnel: w463 -> [w471 w478]
          disable-tunnel: [w476 w482] -> w461
          disable-tunnel: [w475 w481] -> w459
          disable-tunnel: [w473 w480] -> w457
          disable-tunnel: w458 -> [w474 w479]
          frame condition #0 {
            n192 = disable-structure shown="Disabled" {
              frame Disabled {
                # "old filter wheel vi"
                n193 = call "Optec IFW3 - Standalone.vi"() -> ()  [unwired: 11 in, 1 out]
              }
              frame Enabled {
              }
            }
            n194 = Bundle By Name(cluster=w474, "SCD Calibration Optics"="Calibration Optics") -> (w473:T20)
            n195 = call "Optec IFW3 - Set Position with Error Handling.vi"("error in"=w471, "SCD Calibration Optics"="Calibration Optics", "Filter Wheel Selector"=T24."Calibration Polarizers") -> ("error out"=w476:errorcluster, "Actual Position (1-9)"=w475:i32)  [unwired: 6 in, 1 out]
          }
          frame condition #1 (active) {
            n196 = Bundle By Name(cluster=w479, "COMP-S Calibration Wheel"="Calibration Wheel") -> (w480:T20)
            n197 = call "CoMP-S Mechanism - FW.vi"("error in (no error)"=w478, "Calibration Polarizer Filters [Dark]"="Calibration Wheel", "Filter Wheel Selector"=T24."Calibration Polarizers") -> ("error out"=w482:errorcluster, "Position"=w481:i32)  [unwired: 5 in, 2 out]
          }
        }
        n198 = Number To Decimal String(number=w459) -> (decimal integer string=w467:string)  [unwired: 1 in]
        n199 = Concatenate Strings("Updated Calibration Wheel to position:" ("data"), "\t", w467) -> (w460:string)
        n200 = call "SCMP - Write log v2.vi"("Error to log"=w461, "data"=w460) -> ("error out"=w462:errorcluster, "Last Log Entry"=w465:string)  [unwired: 7 in, 1 out]
      }
      frame "AISAS Motors on/off" {
        n201 = Unbundle By Name(w487) -> ("Peripherals"=w489:T15)
        n202 = Select(t="on" ("data"), s="Motors", f="off" ("data")) -> (s? t:f=w494:string)
        n203 = call "Mech on_off.vi"("Peripherals in"=w489, "error in (no error)"=w492, "Motors"="Motors") -> ("error out"=w499:errorcluster, "auto off log"=w484:string, "Peripherals out"=w488:T15)  [unwired: 6 in]
        n204 = Bundle By Name(cluster=w487, "Peripherals"=w488) -> (w486:T20)
        n205 = Concatenate Strings("AISAS Motors " ("data"), w494, w484) -> (w493:string)
        n206 = call "SCMP - Write log v2.vi"("Error to log"=w499, "data"=w493) -> ("error out"=w491:errorcluster, "Last Log Entry"=w490:string)  [unwired: 7 in, 1 out]
      }
      frame "AISAS Move" {
        n207 = Unbundle By Name(w518) -> ("Peripherals.AISAS Mech.lvclass"=w516:refnum<class "AISAS Mech.lvclass">)
        n208 = call "Move.vi"("error in (no error)"=w517, "AISAS Mech in"=w516) -> ("error out"=w515:errorcluster, "AISAS Mech out"=w513:refnum<class "AISAS Mech.lvclass">)  [unwired: 7 in, 1 out]
        n209 = Bundle By Name(cluster=w518, "Peripherals.AISAS Mech.lvclass"=w513) -> (w507:T20)
        n210 = call "Read value.vi"("error in (no error)"=w515, "AISAS Mech in"=w513) -> ("error out"=w514:errorcluster, "Rotation"=w506:T11, "Focus"=w505:T5, "Diffuser"=w509:T10, "Motor"=w508:T23, "Value (String)"=w510:string, "Motor (String)"=w512:string)  [unwired: 3 in]
        n211 = Concatenate Strings("AISAS " ("data"), w512, " set to: " ("data"), w510) -> (w520:string)
        n212 = call "SCMP - Write log v2.vi"("Error to log"=w514, "data"=w520) -> ("error out"=w503:errorcluster, "Last Log Entry"=w519:string)  [unwired: 7 in, 1 out]
        n213 = case shown="\"Rotation\"" w508 {
          tunnel: w509 -> [w524 _ _]
          tunnel: w507 -> [w525 w528 w531]
          tunnel: w505 -> [_ w527 _]
          tunnel: w506 -> [_ _ w530]
          tunnel: [w523 w526 w529] -> w501
          frame "Diffuser " {
            n214 = Bundle By Name(cluster=w525, "Light Shapping Diffuser"=w524) -> (w523:T20)
          }
          frame "Focus" {
            n215 = Bundle By Name(cluster=w528, "Objective Lens Position (mm)"=w527) -> (w526:T20)
          }
          frame "Rotation" {
            n216 = Bundle By Name(cluster=w531, "FOV Rotation (deg)"=w530) -> (w529:T20)
          }
        }
        n217 = call "SCMP write init xml.vi"("error in (no error)"=w503, "FITS Header In"=w501) -> ("error out"=w502:errorcluster)  [unwired: 8 in, 1 out]
      }
      frame "Move AISAS Mechanisms" {
        n218 = disable-structure shown="Disabled" {
          disable-tunnel: [Main_Program_States."Wait for Event" ("Next State") Main_Program_States."Wait for Event" ("Next State")] -> w538
          disable-tunnel: [w551 _] -> w537
          disable-tunnel: [w550 w584] -> w535
          disable-tunnel: [w549 w585] -> w534
          disable-tunnel: w533 -> [w548 w584]
          disable-tunnel: w532 -> [w544 w585]
          frame Disabled {
            n219 = local read "Motors"() -> (w543:bool)
            n220 = call "SCMP - cmp instr val.vi"("FITS Header in"=w544, "Diffuser"="Diffuser 2", "error in (no error)"=w548, "Occulter size"="Size 2", "Rotation"="Rotation [deg] 2", "Focus"="Focus 2") -> ("error out"=w547:errorcluster, "value changed arr"=w545:bool[], "value changed"=w546:bool)  [unwired: 2 in]
            n221 = case shown="True" w546 {
              tunnel: ["" ("Entire Log File") w574] -> w551
              tunnel: [w555 w580] -> w550
              tunnel: [w554 w577] -> w549
              tunnel: w547 -> [w555 w573]
              tunnel: w544 -> [w554 w575]
              tunnel: "Diffuser 2" -> [_ w562]
              tunnel: "Focus 2" -> [_ w569]
              tunnel: "Rotation [deg] 2" -> [_ w568]
              tunnel: "Size 2" -> [_ w564]
              tunnel: w545 -> [_ w571]
              tunnel: w544 -> [_ w563]
              tunnel: w543 -> [_ w558]
              frame False {
              }
              frame True {
                w578 = "\t"
                n222 = call "SCMP -Move AISAS.vi"("FITS Header in"=w563, "Motors"=w558, "Diffuser in"=w562, "error in (no error)"=w573, "value changed arr"=w571, "Rotation in"=w568, "Focus in"=w569) -> ("error out"=w572:errorcluster, "New Rotation"=w559:dbl, "New Focus"=w560:T5, "New Diffuser"=w561:T10)  [unwired: 1 in]
                n223 = local write "Diffuser"(w561) -> ()
                n224 = local write "Focus"(w560) -> ()
                n225 = local write "Rotation [deg]"(w559) -> ()
                n226 = call "SCMP - update instr val.vi"("FITS Header in"=w575, "Diffuser"=w561, "error in (no error)"=w572, "Occulter size"=w564, "Rotation [deg]"=w559, "Focus"=w560) -> ("error out"=w576:errorcluster, "FITS Header out"=w577:T14)  [unwired: 4 in]
                n227 = call "SCMP write init xml.vi"(7:w561, "error in (no error)"=w576, 9:w564, 10:w559, "FITS Header In"=w560) -> ("error out"=w579:errorcluster)  [unwired: 5 in, 1 out]
                n228 = Number To Decimal String(number=w561) -> (decimal integer string=w581:string)  [unwired: 1 in]
                n229 = Number To Fractional String(number=w560, precision (6)=i16 2) -> (F-format string=w570:string)  [unwired: 2 in]
                n230 = Number To Fractional String(number=w559, precision (6)=i16 1) -> (F-format string=w566:string)  [unwired: 2 in]
                n231 = Number To Fractional String(number=w564, precision (6)=i16 2) -> (F-format string=w565:string)  [unwired: 2 in]
                n232 = Concatenate Strings("Instrument set to (Diff/Foc/Rot/Occ):" ("string"), w578, w581, w578, w570, w578, w566, w578, w565, w578) -> (w582:string)
                n233 = call "SCMP - Write log v2.vi"("Error to log"=w579, "data"=w582) -> ("error out"=w580:errorcluster, "Last Log Entry"=w574:string)  [unwired: 7 in, 1 out]
              }
            }
          }
          frame Enabled {
          }
        }
      }
      frame "Change Camera Stage Position" {
        n234 = Build Array("PI cam1 (mm)", "PI cam2 (mm)", "PI cam3 (mm)") -> (w594:T3[])
        n235 = call "SCMP - Control PI Stage Position2.vi"("error in"=w600, "Absolute (F) or \nRelative (T) Move"=FALSE ("Absolute (F) or \nRelative (T) Move"), "set values"=w594) -> ("error out"=w595:errorcluster, "PI set?"=w591:bool, "Position"=w592:dbl[])  [unwired: 6 in]
        n236 = case shown="True" w591 {
          tunnel: ["" w616] -> w601
          tunnel: w590 -> [w603 w615]
          tunnel: [w603 w614] -> w597
          tunnel: [w604 w613] -> w596
          tunnel: w595 -> [w604 w606]
          tunnel: w592 -> [_ w605]
          frame False {
          }
          frame True {
            n237 = Bundle By Name(cluster=w615, "Camera PI (mm)"=w605) -> (w614:T20)
            n238 = Number To Fractional String(number=w605, width (-)=i16 6, precision (6)=i16 2) -> (F-format string=w611:string[])  [unwired: 1 in]
            n239 = Concatenate Strings("Camera Moved to Positon:" ("Recent Log"), w611, "\n" ("string")) -> (w610:string)
            n240 = call "SCMP - Write log v2.vi"("Error to log"=w606, "data"=w610) -> ("error out"=w613:errorcluster, "Last Log Entry"=w616:string)  [unwired: 7 in, 1 out]
          }
        }
      }
      frame "Change Camera Exposure" {
        n241 = local read "Exposure (s)"() -> (w619:dbl)
        n242 = for {
          shift-right: [w631] -> w621
          shift-left: w623 -> [w632]
          tunnel: w618 -> [w634] mode=indexing
          tunnel: w619 -> [w630]
          tunnel: [w630] -> w620
          n243 = Unbundle By Name(w634) -> ("Handle"=w633:i32)
          n244 = call <userlib>:"AT Set Float A.vi"("error in (no error)"=w632, "Value"=w630, "Feature"="ExposureTime", "Hndl"=w633) -> ("error out"=w631:errorcluster)  [unwired: 6 in, 1 out]
        }
        n245 = Number To Fractional String(number=w620) -> (F-format string=w627:string)  [unwired: 3 in]
        n246 = Concatenate Strings("Camera Exposure Changed to " ("data"), w627, " seconds" ("string")) -> (w625:string)
        n247 = call "SCMP - Write log v2.vi"("Error to log"=w621, "data"=w625) -> ("error out"=w622:errorcluster, "Last Log Entry"=w624:string)  [unwired: 7 in, 1 out]
      }
      frame "Set Camera AOI" {
        n248 = disable-structure shown="Enabled" {
          disable-tunnel: w646 -> [w652 w657]
          disable-tunnel: "Binning" -> [w651 w656]
          disable-tunnel: [w650 w655] -> w640
          disable-tunnel: w638 -> [w649 w654]
          disable-tunnel: [w648 w653] -> w637
          frame Disabled {
            n249 = call "Andor Neo - Set Binning v2.vi"("Andor Neo"=w649, "error in"=w652, "Binning"=w651) -> ("error out"=w650:errorcluster, "Andor Neo out"=w648:T17[])  [unwired: 7 in]
          }
          frame Enabled {
            n250 = for {
              tunnel: w656 -> [w660]
              shift-right: [w659] -> w655
              shift-left: w657 -> [w662]
              tunnel: w654 -> [w661] mode=indexing
              tunnel: [w658] -> w653 mode=indexing
              n251 = call "Andor Neo - Set Binning subvi.vi"("error in"=w662, "Binning"=w660, "Andor"=w661) -> ("error out"=w659:errorcluster, "Andor out"=w658:T17)  [unwired: 7 in]
            }
          }
        }
        n252 = property on="Binning" class="Enum (strict)"() -> ("RingText.Text"=w639:string)  [unwired: 2 in, 2 out]
        n253 = Concatenate Strings("Set Camera Binning: " ("Recent Log"), w639) -> (w644:string)
        n254 = call "SCMP - Write log v2.vi"("Error to log"=w640, "data"=w644) -> ("error out"=w641:errorcluster, "Last Log Entry"=w643:string)  [unwired: 7 in, 1 out]
      }
      frame "Andor Adv Settings" {
        n255 = Index Array(array=w664) -> (element #1=w667:T17, element #2=w666:T17)  [unwired: 2 in]
        n256 = Unbundle By Name(w667) -> ("Handle"=w670:i32)
        n257 = Unbundle By Name(w666) -> ("Handle"=w671:i32)
        n258 = call-by-ref "SCMP Andor setupdialog.vi"(error in=w669, "Handle 2"=w671, "Handle"=w670) -> (error out=w668:errorcluster)  [unwired: 10 in, 2 out]
      }
      frame "Stop" {
        n259 = Unbundle By Name(w675) -> ("Peripherals.PI Stages"=w674:bool)
        n260 = global read "Global demo.vi" "demo"() -> (w678:bool)
        n261 = Not(x=w678) -> (.not. x?=w676:bool)
        n262 = Compound Arithmetic op=AND(w676, w672, w674) -> (w677:bool)
        n263 = case shown="True" w677 {
          tunnel: [FALSE w688] -> w679
          frame False {
          }
          frame True {
            n264 = Two Button Dialog(message="Set PI stages to parking position?", 1:"No" ("F button name (\"Cancel\")"), 2:"Yes" ("T button name (\"OK\")")) -> (T button?=w688:bool)
          }
        }
        n265 = case shown="True" w679 {
          tunnel: w682 -> [w693 w702]
          tunnel: [w693 w701] -> w681
          tunnel: ["Main Loop Terminated" ("data") w698] -> w680
          frame False {
          }
          frame True {
            w699 = "\n" ("string")
            n266 = disable-structure shown="SCMP==COMP, Default" {
              disable-tunnel: [w709 w710] -> w703
              frame condition #0 (active) {
                n267 = global read "Globals.vi" "comp parking pos"() -> (w709:dbl[])
              }
              frame condition #1 {
                n268 = global read "Globals.vi" "scd parking pos"() -> (w710:dbl[])
              }
            }
            n269 = call "SCMP - Control PI Stage Position2.vi"("error in"=w702, "Absolute (F) or \nRelative (T) Move"=FALSE ("Absolute (F) or \nRelative (T) Move"), "set values"=w703) -> ("error out"=w701:errorcluster, "Position"=w697:dbl[])  [unwired: 6 in, 1 out]
            n270 = Index Array(array=w697) -> (element #1=w694:dbl, element #2=w695:dbl, element #3=w696:dbl)  [unwired: 3 in]
            n271 = Number To Fractional String(number=w697, width (-)=i16 6, precision (6)=i16 2) -> (F-format string=w707:string[])  [unwired: 1 in]
            n272 = local write "PI cam1 (mm)"(w694) -> ()
            n273 = local write "PI cam2 (mm)"(w695) -> ()
            n274 = local write "PI cam3 (mm)"(w696) -> ()
            n275 = Concatenate Strings("Camera Moved to Positon:" ("Recent Log"), w707, w699, "Main Loop Terminated" ("data"), w699) -> (w698:string)
          }
        }
        n276 = call "SCMP - Write log v2.vi"("Error to log"=w681, "data"=w680) -> ("error out"=w683:errorcluster, "Last Log Entry"=w685:string)  [unwired: 7 in, 1 out]
      }
    }
    "FITS Header" <- w90
    "Andor Neo" <- w91
    n277 = Not(x=w87) -> (.not. x?=→"Main Loop":bool)
    n278 = local write "Main Loop Error"(w92) -> ()
    n279 = Concatenate Strings(w97, w98) -> (w96:string)
    "Latest Actions" <- w96
    n280 = call <vilib>:"General Error Handler.vi"("error in (no error)"=w92) -> ("error out"=w93:errorcluster)  [unwired: 10 in, 4 out]
    n281 = call <vilib>:"Clear Errors.vi"("error in (no error)"=w93) -> ("error out"=w95:errorcluster)  [unwired: 5 in, 1 out]
  }
  n282 = while {
    shift-right: [w715] -> _
    shift-left: w11 -> [w712]
    tunnel: [w722] -> w35
    shift-right: [w719] -> _
    shift-left: 0.0 ("Time Target (s)") -> [w717]
    shift-right: [w713] -> w18
    shift-left: w19 -> [w716]
    stop <- w721 stop-if-true
    n283 = call "Elapsed Time"("Time Target (s)"=w717, "error in (no error)"=w712) -> ("Time has Elapsed"=w720:bool, "error out"=w711:errorcluster)  [unwired: 10 in, 6 out]
    n284 = case shown="True" w720 {
      tunnel: w711 -> [w724 w730]
      tunnel: [w724 w729] -> w714
      tunnel: w717 -> [w725 _]
      tunnel: [w725 w728] -> w719
      tunnel: w716 -> [w723 w727]
      tunnel: [w723 w726] -> w713
      frame False {
      }
      frame True {
        w728 = 10.0  # Log cadence time [s]
        n285 = stacked-sequence {
          frame #0 {
            n286 = local write "Log Loop"(FALSE ("Log Loop")) -> ()
            n287 = Wait (ms)(milliseconds to wait=u32 200) -> ()  [unwired: 1 out]
          }
          frame #1 {
            n288 = local write "Log Loop"(TRUE ("Log Loop")) -> ()
          }
        }
        n289 = case shown="True" "Enable Data Logging" {
          tunnel: w730 -> [w736 w748]
          tunnel: [w736 w743] -> w729
          tunnel: w727 -> [w735 w739]
          tunnel: [w735 w745] -> w726
          frame False {
          }
          frame True {
            n290 = call "Read Zone Temps v2.vi"("Peripherals"=w739, "error in"=w748) -> ("error out"=w738:errorcluster, "Air Temp [C]"=w737:dbl, "Camera Body [C]"=w749:sgl, "Pre-Filter Temp [C}"=w746:sgl, "Peripherals out"=w744:T15)  [unwired: 5 in]
            "Air around Camera [C]" <- w749
            "Air around \nprefilter wheel [C]" <- w746
            "Air around Lyot Filter [C]" <- w737
            n291 = call "ILX Status.vi"("Peripherals in"=w744, "error in"=w738) -> ("error out"=w747:errorcluster, "Temperature"=w750:dbl, "Peripherals out"=w745:T15)  [unwired: 4 in, 3 out]
            "Lyot Filter Temp [C]" <- w750
            n292 = local read "Camera 1 Temp [C}"() -> (w742:dbl)
            n293 = Build Array(w750, w746, w749, w737, w742) -> (w741:dbl[])
            n294 = disable-structure shown="SCMP==COMP, Default" {
              disable-tunnel: w741 -> [w752 w754]
              disable-tunnel: [w751 w754] -> w740
              frame condition #0 (active) {
                n295 = local read "Camera 2 Temp [C}"() -> (w753:dbl)
                n296 = Build Array (concatenate)(w752, w753) -> (w751:dbl[])
              }
              frame condition #1 {
              }
            }
            n297 = call "SCMP - Write Eng Data v2.vi"("error in"=w747, "Temp Data"=w740) -> ("error out"=w743:errorcluster)  [unwired: 6 in, 3 out]
            "Eng Data Error" <- w743
          }
        }
      }
    }
    n298 = local read "Main Loop"() -> (w722:bool)
    n299 = Not(x=w722) -> (.not. x?=w721:bool)
    n300 = Wait (ms)(milliseconds to wait=u32 100) -> ()  [unwired: 1 out]
    n301 = call <vilib>:"Clear Errors.vi"("error in (no error)"=w714) -> ("error out"=w715:errorcluster)  [unwired: 5 in, 1 out]
  }
  "Log Loop" <- w35
  n302 = Unbundle By Name(w18) -> ("Zone temp ref"=w3:variant)
  n303 = disable-structure shown="Disabled" {
    frame Disabled {
      (unwired) string[] ["Cookbook Stopped"] ("[user-defined descriptions]")
      w756 = T25 2 items=["no dialog", "OK message", "continue or stop message", "OK message + warnings", "continue/stop + warnings"] ("type of dialog (OK msg:1)")
      n304 = call <vilib>:"General Error Handler.vi"("[user-defined codes]"=i32[] [5000], "type of dialog (OK msg:1)"=w756) -> ("[user-defined descriptions]"=w758:string[])  [unwired: 8 in, 5 out]
      n305 = One Button Dialog(message="Please Enter \nAn Observer\nAnd A Comment") -> ()  [unwired: 1 in, 1 out]
    }
    frame Enabled {
    }
  }
  n306 = Variant To Data(type=refnum<k24> refnum ("ILabVIEW In"), Variant=w3) -> (data=w2:refnum<k24>)  [unwired: 1 in, 1 out]
  n307 = Not A Number/Path/Refnum?(number/path/refnum=w2) -> (NaN/Path/Refnum?=w1:bool)
  n308 = case shown="False" w1 {
    tunnel: [w760 errorcluster {"status"=FALSE, "code"=0, "source"=""} ("error out")] -> w32
    tunnel: w2 -> [w759 _]
    frame False {
      n309 = call "Std_Bus_Close_System.vi"("ILabVIEW In"=w759) -> ("error out"=w760:errorcluster)  [unwired: 1 in, 17 out]
    }
    frame True {
    }
  }
  n310 = call "SCMP Andor Neo Close.vi"("error in (no error)"=w33, "Andor Neo"=w25) -> ("error out"=w36:errorcluster)  [unwired: 9 in]
  n311 = Merge Errors(w36, w32) -> (w28:errorcluster)
  n312 = Unbundle By Name(w28) -> ("status"=w29:bool)
  n313 = call "SCMP - Write log v2.vi"("Error to log"=w28, "data"="Program Ended") -> ("error out"=→"Main Loop Error":errorcluster)  [unwired: 7 in, 2 out]
  n314 = And(x=FALSE, y=w29) -> (x .and. y?=→"Program":bool)
  "Instrument" <- w5
